vi "Autonomous Independent.vi"() -> ()   [LabVIEW 2016]
doc: "This VI is called when autonomous begins, and will automatically be terminated when autonomous ends. You can carry out timed or sensor driven robot movement independently without needing to return to the caller."
uses:
  <vilib>/Rock Robotics/WPI/Relay/WPI_RelayValue.ctl
  <vilib>/Rock Robotics/WPI/Utilities/WPI_GetSetVariantRefNum.vi
  <vilib>/Rock Robotics/Network Tables/NT Read String.vi
  <vilib>/Rock Robotics/Network Tables/NT Write Numeric Array.vi
  Robot Global Data.vi
  <vilib>/Rock Robotics/WPI/RobotDrive/WPI_RobotDriveArcadeDrive_Standard(NoSaturation).vi
  <vilib>/Rock Robotics/WPI/RobotDrive/WPI_RobotDriveArcadeDrive_RatioCurve.vi
panel:
  out "time up? 16":bool
  out "time up? 15":bool
  out "time up? 14":bool
  out "time up? 13":bool
  out "time up? 12":bool
  out "time up? 11":bool
  out "time up? 10":bool
  out "time up? 9":bool
  out "time up? 8":bool
  out "time up? 7":bool
  out "time up? 6":bool
  out "time up? 5":bool
  out "time up? 4":bool
  out "time up? 3":bool
  in  "Base 2":dbl=0.6
  in  "Tolerance 2":dbl=0.08
  in  "Ratio 2":dbl=0.25 format="%#_13g"
  out "time up? 2":bool
  out "time up?":bool
  in  "Ratio":dbl=0.25 format="%#_13g"
  in  "Tolerance":dbl=0.08
  in  "Base":dbl=0.6
  # "Be sure to right-click and choose Data Operations>>Make Current Value default if you want to save the array values with the VI"
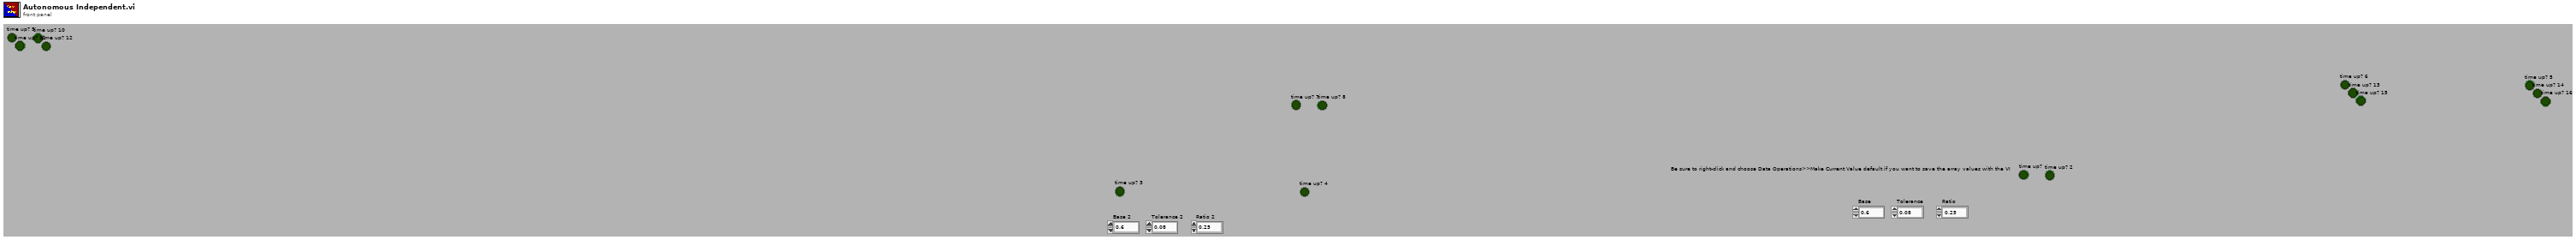
[diagram p1: front panel]
types:
  T1 = typedef "WPI_JoystickDevRef.ctl" = cluster{"Device":T2}
  T2 = typedef "WPI_JoystickDeviceEnum.ctl" = enum16{"USB 0", "USB 1", "USB 2", "USB 3", "USB 4", "USB 5"}
  T3 = typedef "WPI_RobotDriveDevRef.ctl" = cluster{"DevStatus":errorcluster, "Motors[]":T4[], "Square Inputs":bool, "Max Output":dbl}
  T4 = typedef "WPI_MotorControlDeviceRef.ctl" = cluster{"DeviceStatus":errorcluster, "Type":T5, "PWM":cluster{"PWM Channel":T6, "DeadBand":T7}, "CAN":cluster{"Device Number":u8, "SetOutput VI Ref":variant, "GetOutput VI Ref":variant, "Enable VI Ref":variant, "Disable VI Ref":variant, "Data":variant}, "Invert":bool}
  T5 = typedef "WPI_MotorControlType.ctl" = enum16{"PWM", "CAN"}
  T6 = typedef "FPGA_DIOPWMChannel.ctl" = enum8{"PWM 0", "PWM 1", "PWM 2", "PWM 3", "PWM 4", "PWM 5", "PWM 6", "PWM 7", "PWM 8", "PWM 9", "PWM MXP 0", "PWM MXP 1", "PWM MXP 2", "PWM MXP 3", "PWM MXP 4", "PWM MXP 5", "PWM MXP 6", "PWM MXP 7", "PWM MXP 8", "PWM MXP 9", "Invalid"}
  T7 = typedef "WPI_PWMDeadband.ctl" = cluster{"Name":string, "maxPositivePwm":i32, "minPositivePwm":i32, "centerPwm":i32, "maxNegativePwm":i32, "minNegativePwm":i32, "angularRange":u16}
  T8 = typedef "WPI_RelayDevRef.ctl" = cluster{"DevStatus":errorcluster, "Relay Channel":T9, "Relay Direction":T10}
  T9 = typedef "FPGA_DIORelayChannel.ctl" = enum8{"Relay 0", "Relay 1", "Relay 2", "Relay 3", "Invalid"}
  T10 = typedef "WPI_RelayDirection.ctl" = enum16{"Both directions", "Forward only", "Reverse only"}
  T11 = typedef "WPI_RelayValue.ctl" = enum16{"Off", "On", "Forward", "Reverse"}
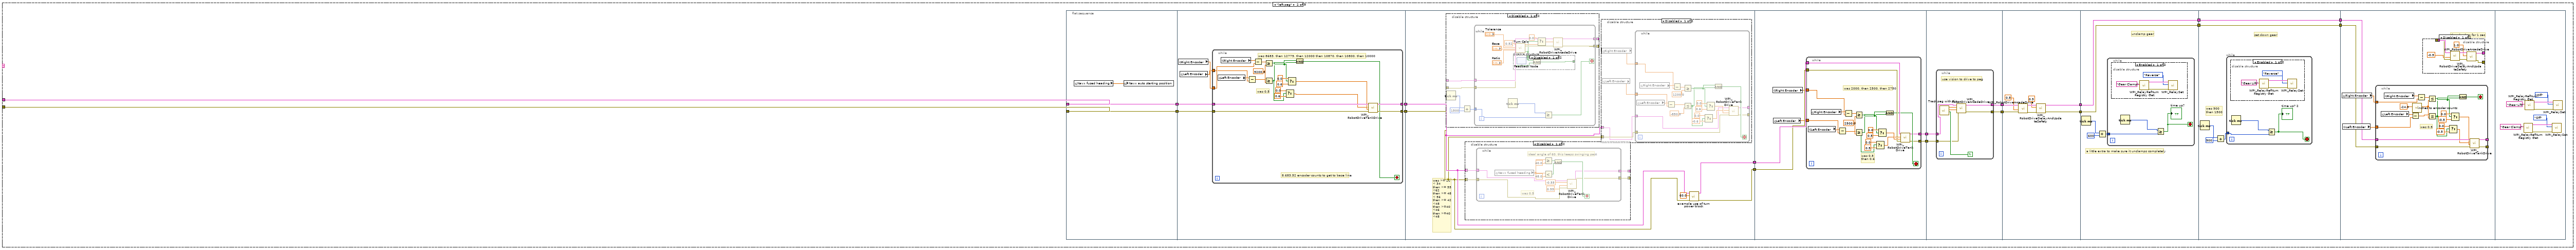
[diagram p3: hidden frame]
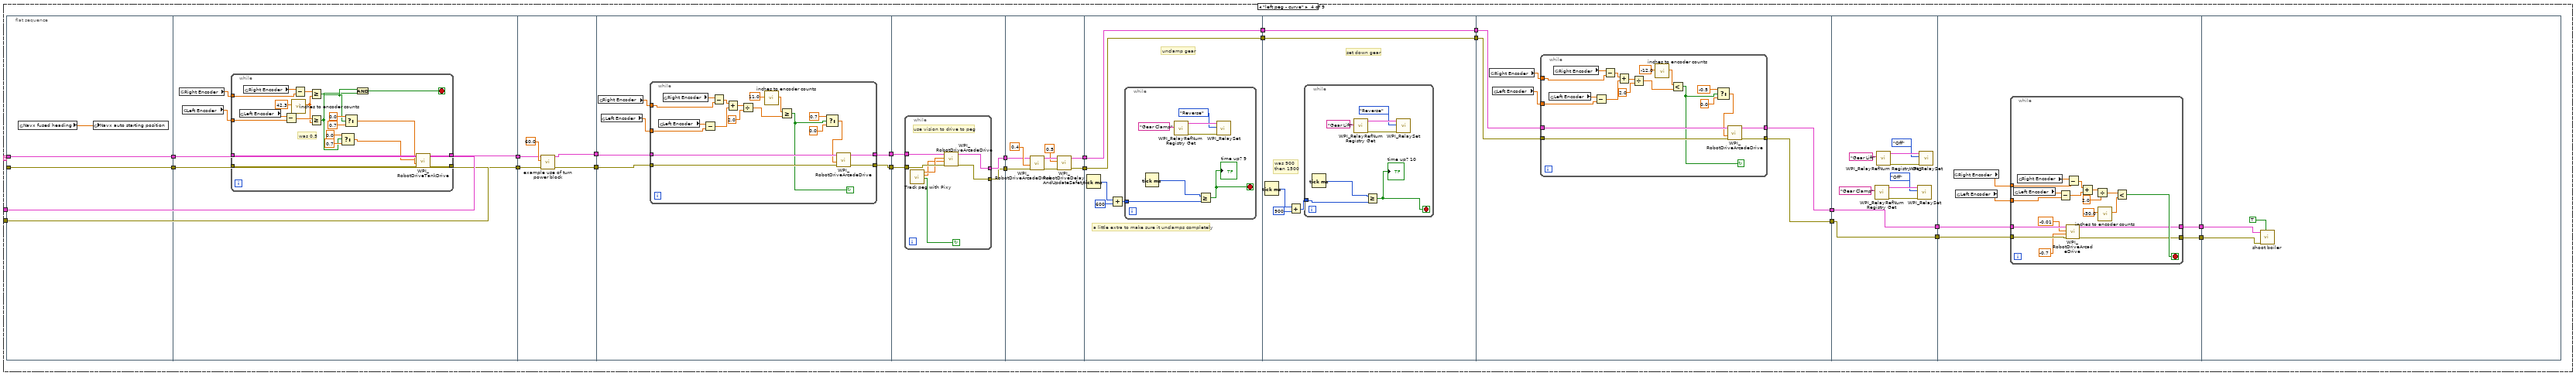
[diagram p14: hidden frame]
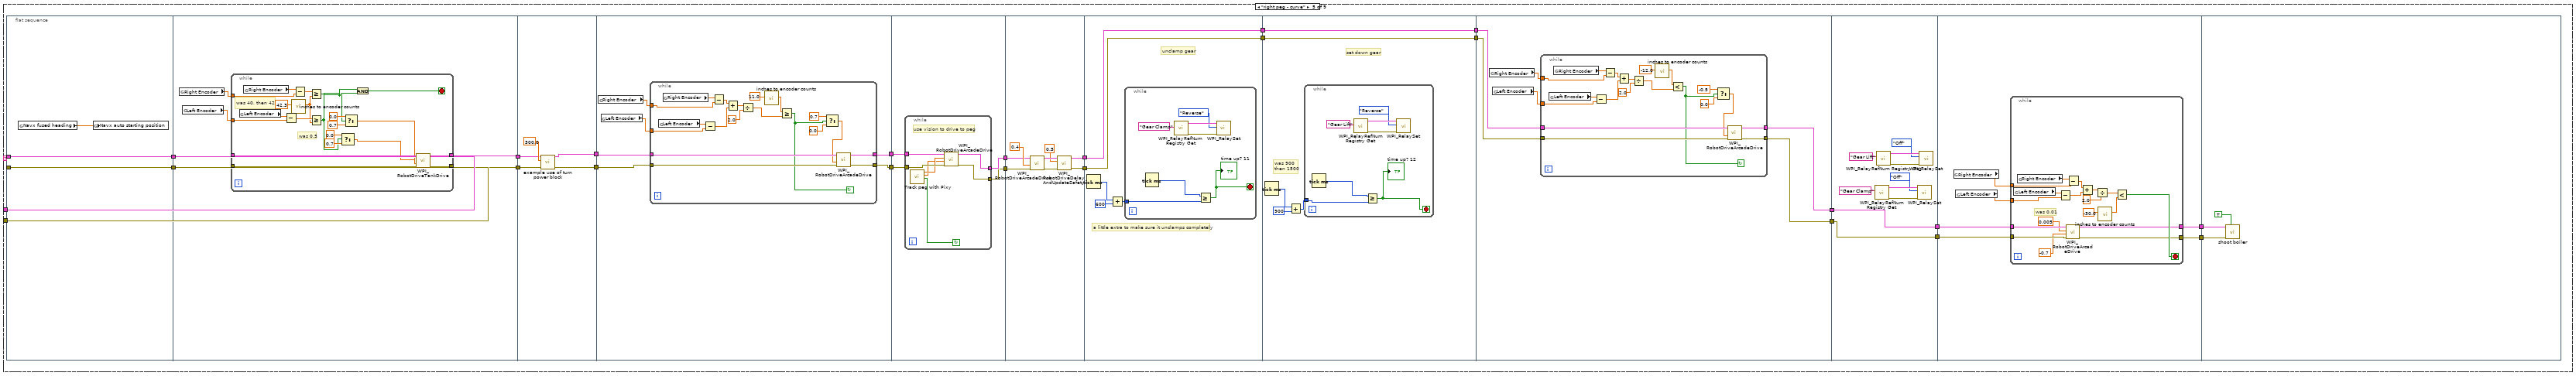
[diagram p15: hidden frame]
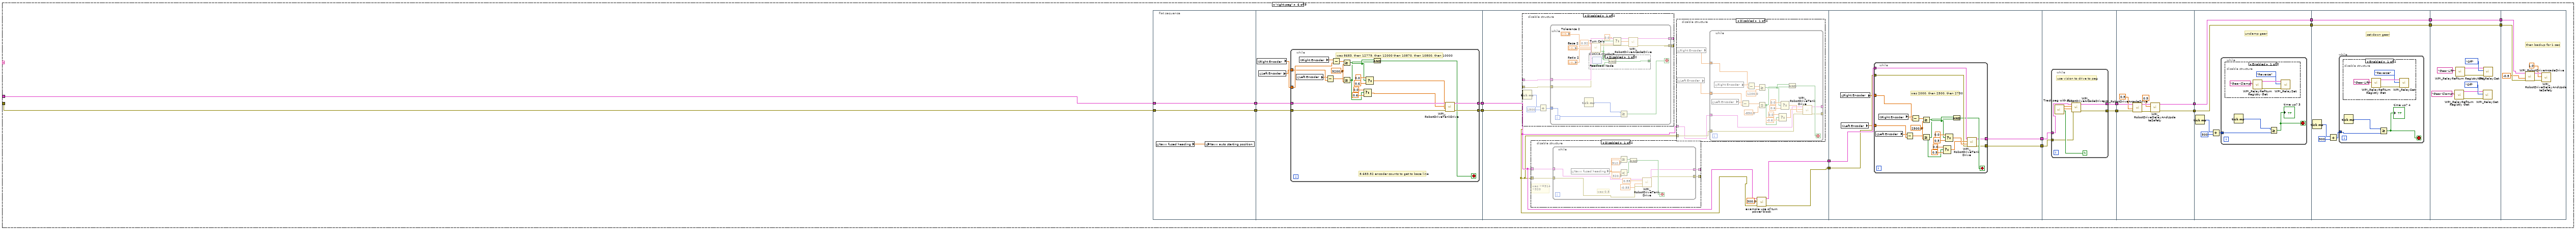
[diagram p16: hidden frame]
diagram:
  (unwired) "This function is run in parallel when the autonomous period begins. It will be terminated automatically when the period ends.\n\nNote that all Driver Station inputs are automatically latched and will not change once auto begins."
  # "This tells you the autonomous selected\nfrom the dashboard"
  # "Every 20ms, report that we are running autonomous\ncode. Loop will abort the same time as the VI."
  # "This gives you the joystick value\nthat is often the throttle"
  # "Use time and/or sensors to control how the robot drives."
  # "This tells you the driver position\nand alliance color"
  n1 = while {
    stop <- FALSE stop-if-true
    n2 = call <vilib>:"WPI_DriverStationReport Robot Code State.vi"("Autonomous"=TRUE) -> ()  [unwired: 10 in, 1 out]
    n3 = Wait (ms)(milliseconds to wait=u32 20) -> ()  [unwired: 1 out]
  }
  n4 = call <vilib>:"WPI_DriverStationGet Alliance Info.vi"() -> ()  [unwired: 12 out]
  n5 = call <vilib>:"WPI_JoystickRefNum Registry Get.vi"("refnum name"="Joystick 0") -> ("JoystickDevRef"=w15:T1)  [unwired: 1 in, 9 out]
  n6 = call <vilib>:"WPI_JoystickGetValues.vi"("JoystickDevRef"=w15) -> ("Axes"=w11:dbl[])  [unwired: 6 in, 4 out]
  n7 = call-poly <vilib>:"NT Read Value.vi"("Name"="Auto Selector") -> ("String"=w12:string)  [unwired: 9 in, 1 out]
  n8 = call-poly <vilib>:"NT Write Value.vi"("Numeric Array"=w11, "Name"="Joystick 0/Axes") -> ()  [unwired: 9 in, 1 out]
  n9 = Index Array(array=w11, index=2) -> ()  [unwired: 1 out]
  n10 = call <vilib>:"WPI_RobotDriveRefNum Registry Get.vi"("refnum name"="Drive") -> ("error out"=w7:errorcluster, "RobotDriveDevRef"=w8:T3)  [unwired: 9 in]
  n11 = call <vilib>:"WPI_RelayRefNum Registry Get.vi"("refnum name"="Ball Stirrer") -> ("error out"=w1:errorcluster, "RelayDevRef"=w2:T8)  [unwired: 9 in]
  n12 = call <vilib>:"WPI_MotorControlRefNum Registry Get.vi"("refnum name"="Shooter") -> ("error out"=w4:errorcluster, "MotorControlDevRef"=w5:T4)  [unwired: 9 in]
  n13 = case shown="\"center peg shoot - right\"" w12 {
    tunnel: w8 -> [_ w37 w257 w490 w679 w861 w1070 w1176 w1339]
    tunnel: w7 -> [_ w36 w256 w489 w678 w860 w1069 w1175 w1338]
    tunnel: w5 -> [_ _ _ _ _ _ _ _ _]
    tunnel: w4 -> [_ _ _ _ _ _ _ _ _]
    tunnel: w2 -> [_ _ _ _ _ _ _ _ _]
    tunnel: w1 -> [_ _ _ _ _ _ _ _ _]
    frame Default {
      # "You can put your main auto here, or you can right-click on the case and make any\nother frame be the default case."
      # "This is the frame that will execute if no selection is made, or if it is not recognized"
    }
    frame "left peg" {
      n14 = flat-sequence {
        tunnel: w36 -> [w39]
        tunnel: w37 -> [w40]
        tunnel: [w40] -> w21
        tunnel: [w39] -> w20
        tunnel: [w44] -> w27
        tunnel: [w43] -> w26
        tunnel: w21 -> [w46]
        tunnel: w20 -> [w45]
        tunnel: [w70] -> w25
        tunnel: w26 -> [w67]
        tunnel: w27 -> [w68]
        tunnel: [w69] -> w24
        tunnel: [w141] -> w35
        tunnel: [w140] -> w34
        tunnel: w25 -> [w143]
        tunnel: w24 -> [w142]
        tunnel: w35 -> [w167]
        tunnel: w34 -> [w166]
        tunnel: [w165] -> w31
        tunnel: [w164] -> w29
        tunnel: w31 -> [w182]
        tunnel: [w176] -> w30
        tunnel: w29 -> [w181]
        tunnel: [w175] -> w28
        tunnel: [w184] -> w33
        tunnel: w30 -> [w184]
        tunnel: [w183] -> w32
        tunnel: w28 -> [w183]
        tunnel: [w196] -> w23
        tunnel: w33 -> [w196]
        tunnel: [w195] -> w22
        tunnel: w32 -> [w195]
        tunnel: w22 -> [w207]
        tunnel: w23 -> [w208]
        frame #0 {
          n15 = global read "Robot Global Data.vi" "Navx fused heading"() -> (w38:dbl)
          n16 = global write "Robot Global Data.vi" "Navx auto starting position"(w38) -> ()
        }
        frame #1 {
          n17 = global read "Robot Global Data.vi" "Right Encoder"() -> (w42:dbl)
          n18 = global read "Robot Global Data.vi" "Left Encoder"() -> (w41:dbl)
          n19 = while {
            tunnel: w46 -> [w66]
            tunnel: w45 -> [w65]
            tunnel: [w57] -> w44
            tunnel: [w56] -> w43
            tunnel: w42 -> [w54]
            tunnel: w41 -> [w51]
            stop <- w49 stop-if-true
            w58 = 9200.0 ("y")
            # "was 0.5"
            # "was 8683, then 12779, then 12000 then 10870, then 10800, then 10000"
            # "8,683.52 encoder counts to get to base line"
            n20 = global read "Robot Global Data.vi" "Left Encoder"() -> (w52:dbl)
            n21 = global read "Robot Global Data.vi" "Right Encoder"() -> (w55:dbl)
            n22 = Subtract(x=w52, y=w51) -> (x-y=w50:dbl)
            n23 = Subtract(x=w55, y=w54) -> (x-y=w53:dbl)
            n24 = Greater Or Equal?(x=w53, y=w58) -> (x >= y?=w60:bool)
            n25 = Greater Or Equal?(x=w50, y=w58) -> (x >= y?=w59:bool)
            n26 = Select(t=0.0, s=w59, f=0.6) -> (s? t:f=w47:dbl)
            n27 = Select(t=0.0, s=w60, f=0.6) -> (s? t:f=w48:dbl)
            n28 = And(x=w60, y=w59) -> (x .and. y?=w49:bool)
            n29 = call <vilib>:"WPI_RobotDriveTankDrive.vi"("error in (no error)"=w65, "Right axis value"=w48, "Left axis value"=w47, "RobotDriveDevRef"=w66) -> ("error out"=w56:errorcluster, "RobotDriveDevRef"=w57:T3)  [unwired: 5 in, 1 out]
          }
        }
        frame #2 {
          # "was >= 28\n< 34\nthen >= 55\n<62\nthen >= 48\n< 56\nthen >= 42\n<48\nthen >=40\n<46\nthen >=40\n<48"
          n30 = disable-structure shown="Disabled" {
            disable-tunnel: _ -> [w119 _]
            disable-tunnel: _ -> [w118 _]
            disable-tunnel: [w117 _] -> _
            disable-tunnel: [w116 _] -> _
            frame Disabled {
              n31 = Tick Count (ms)() -> (millisecond timer value=w114:u32)
              n32 = Add(x=w114, y=u32 1500) -> (x+y=w113:u32)
              n33 = while {
                tunnel: w119 -> [w134]
                tunnel: w118 -> [w133]
                tunnel: [w124] -> w117
                tunnel: [w123] -> w116
                tunnel: w113 -> [w120]
                stop <- w121 stop-if-true
                n34 = Tick Count (ms)() -> (millisecond timer value=w122:u32)
                n35 = call "Turn Calc.vi"("Desired Angle (radians)"=0.52, "Tolerance"="Tolerance", "Base"="Base", "Ratio"="Ratio") -> ("Drive X Output"=w126:dbl, "In Range?"=w125:bool)  [unwired: 12 in, 2 out]
                n36 = disable-structure shown="Disabled" {
                  disable-tunnel: w125 -> [w136 _]
                  disable-tunnel: [w135 _] -> _
                  frame Disabled {
                    n37 = feedback #1() -> (w137:bool)  [unwired: 1 in]
                    n38 = feedback-in #1(w136) -> ()
                    n39 = And(x=w136, y=w137) -> (x .and. y?=w135:bool)
                  }
                  frame Enabled {
                  }
                }
                n40 = Select(t=0.0 ("f"), s=w125, f=w126) -> (s? t:f=w128:dbl)
                n41 = Greater Or Equal?(x=w122, y=w120) -> (x >= y?=w121:bool)
                n42 = call-poly <vilib>:"WPI_RobotDriveArcadeDrive.vi"("error in (no error)"=w133, "X axis value"=w128, "RobotDriveDevRef"=w134) -> ("error out"=w123:errorcluster, "RobotDriveDevRef"=w124:T3)  [unwired: 6 in, 1 out]
              }
            }
            frame Enabled {
            }
          }
          n43 = disable-structure shown="Disabled" {
            disable-tunnel: w67 -> [w75 _]
            disable-tunnel: w68 -> [w74 _]
            disable-tunnel: [w73 _] -> _
            disable-tunnel: [w72 _] -> _
            frame Disabled {
              n44 = while {
                tunnel: w74 -> [w76]
                tunnel: w75 -> [w80]
                tunnel: [w82] -> w73
                tunnel: [w81] -> w72
                stop <- w83 stop-if-true
                # "ideal angle of 60, this keeps swinging past"
                # "was 0.5"
                n45 = global read "Robot Global Data.vi" "Navx fused heading"() -> (w79:dbl)
                n46 = Greater Or Equal?(x=w79, y=40.0) -> (x >= y?=w85:bool)
                n47 = Less?(x=w79, y=48.0) -> (x < y?=w84:bool)
                n48 = And(x=w85, y=w84) -> (x .and. y?=w83:bool)
                n49 = call <vilib>:"WPI_RobotDriveTankDrive.vi"("error in (no error)"=w80, "Right axis value"=0.55, "Left axis value"=-0.55 ("x"), "RobotDriveDevRef"=w76) -> ("error out"=w81:errorcluster, "RobotDriveDevRef"=w82:T3)  [unwired: 5 in, 1 out]
              }
            }
            frame Enabled {
            }
          }
          n50 = disable-structure shown="Disabled" {
            disable-tunnel: w67 -> [w91 _]
            disable-tunnel: w68 -> [w90 _]
            frame Disabled {
              n51 = global read "Robot Global Data.vi" "Right Encoder"() -> (w88:dbl)
              n52 = global read "Robot Global Data.vi" "Left Encoder"() -> (w89:dbl)
              n53 = while {
                tunnel: w88 -> [w101]
                tunnel: w89 -> [w100]
                tunnel: [w96] -> _
                tunnel: [w95] -> _
                tunnel: w90 -> [w93]
                tunnel: w91 -> [w92]
                stop <- w97 stop-if-true
                n54 = global read "Robot Global Data.vi" "Left Encoder"() -> (w103:dbl)
                n55 = global read "Robot Global Data.vi" "Right Encoder"() -> (w105:dbl)
                n56 = Subtract(x=w103, y=w100) -> (x-y=w102:dbl)
                n57 = Subtract(x=w105, y=w101) -> (x-y=w104:dbl)
                n58 = Greater Or Equal?(x=w104, y=1200.0) -> (x >= y?=w108:bool)
                n59 = Less Or Equal?(x=w102, y=-850.0) -> (x <= y?=w107:bool)
                n60 = Select(t=0.0, s=w107, f=-0.6) -> (s? t:f=w98:dbl)
                n61 = Select(t=0.0, s=w108, f=0.6) -> (s? t:f=w99:dbl)
                n62 = And(x=w108, y=w107) -> (x .and. y?=w97:bool)
                n63 = call <vilib>:"WPI_RobotDriveTankDrive.vi"("error in (no error)"=w92, "Right axis value"=w99, "Left axis value"=w98, "RobotDriveDevRef"=w93) -> ("error out"=w95:errorcluster, "RobotDriveDevRef"=w96:T3)  [unwired: 5 in, 1 out]
              }
            }
            frame Enabled {
            }
          }
          n64 = call "example use of turn power block.vi"("error in (no error)"=w67, "desired angle"=60.0, "RobotDriveDevRef"=w68) -> ("error out"=w69:errorcluster, "RobotDriveDevRef 2"=w70:T3)  [unwired: 7 in]
        }
        frame #3 {
          n65 = global read "Robot Global Data.vi" "Right Encoder"() -> (w139:dbl)
          n66 = global read "Robot Global Data.vi" "Left Encoder"() -> (w138:dbl)
          n67 = while {
            tunnel: w139 -> [w152]
            tunnel: w138 -> [w151]
            tunnel: w143 -> [w148]
            tunnel: w142 -> [w147]
            tunnel: [w145] -> w141
            tunnel: [w144] -> w140
            stop <- w146 stop-if-true
            w157 = 2500.0 ("y")
            # "was 0.5\nthen 0.6"
            # "was 2000, then 2500, then 2750"
            n68 = global read "Robot Global Data.vi" "Left Encoder"() -> (w154:dbl)
            n69 = global read "Robot Global Data.vi" "Right Encoder"() -> (w156:dbl)
            n70 = Subtract(x=w154, y=w151) -> (x-y=w153:dbl)
            n71 = Subtract(x=w156, y=w152) -> (x-y=w155:dbl)
            n72 = Greater Or Equal?(x=w155, y=w157) -> (x >= y?=w159:bool)
            n73 = Greater Or Equal?(x=w153, y=w157) -> (x >= y?=w158:bool)
            n74 = Select(t=0.0, s=w158, f=0.5) -> (s? t:f=w149:dbl)
            n75 = Select(t=0.0, s=w159, f=0.5) -> (s? t:f=w150:dbl)
            n76 = And(x=w159, y=w158) -> (x .and. y?=w146:bool)
            n77 = call <vilib>:"WPI_RobotDriveTankDrive.vi"("error in (no error)"=w147, "Right axis value"=w150, "Left axis value"=w149, "RobotDriveDevRef"=w148) -> ("error out"=w144:errorcluster, "RobotDriveDevRef"=w145:T3)  [unwired: 5 in, 1 out]
          }
        }
        frame #4 {
          n78 = while {
            tunnel: w167 -> [w168]
            tunnel: w166 -> [w169]
            tunnel: [w171] -> w165
            tunnel: [w170] -> w164
            stop <- w172 continue-if-true
            # "use vision to drive to peg"
            n79 = call "Track peg with Pixy.vi"() -> ("sees peg"=w172:bool, "y output"=w173:dbl, "x output"=w174:dbl)  [unwired: 8 in]
            n80 = call-poly <vilib>:"WPI_RobotDriveArcadeDrive.vi"("error in (no error)"=w169, "Y axis value"=w173, "X axis value"=w174, "RobotDriveDevRef"=w168) -> ("error out"=w170:errorcluster, "RobotDriveDevRef"=w171:T3)  [unwired: 5 in, 1 out]
          }
        }
        frame #5 {
          n81 = call-poly <vilib>:"WPI_RobotDriveArcadeDrive.vi"("error in (no error)"=w181, "Y axis value"=0.5, "RobotDriveDevRef"=w182) -> ("error out"=w179:errorcluster, "RobotDriveDevRef"=w180:T3)  [unwired: 6 in, 1 out]
          n82 = call <vilib>:"WPI_RobotDriveDelayAndUpdateSafety.vi"("error in (no error)"=w179, "Delay (s)"=0.5, "RobotDriveDevRef"=w180) -> ("error out"=w175:errorcluster, "RobotDriveDevRef 2"=w176:T3)  [unwired: 7 in]
        }
        frame #6 {
          # "a little extra to make sure it unclamps completely"
          # "unclamp gear"
          n83 = Tick Count (ms)() -> (millisecond timer value=w186:u32)
          n84 = Add(x=w186, y=u32 600) -> (x+y=w185:u32)
          n85 = while {
            tunnel: w185 -> [w188]
            stop <- w189 stop-if-true
            n86 = disable-structure shown="Enabled" {
              frame Enabled {
                n87 = call <vilib>:"WPI_RelayRefNum Registry Get.vi"("refnum name"="Gear Clamp") -> ("error out"=w193:errorcluster, "RelayDevRef"=w194:T8)  [unwired: 9 in]
                n88 = call <vilib>:"WPI_RelaySet.vi"("error in (no error)"=w193, "RelayValue"=WPI_RelayValue."Reverse", "RelayDevRef"=w194) -> ()  [unwired: 7 in, 2 out]
              }
              frame Disabled {
              }
            }
            n89 = Tick Count (ms)() -> (millisecond timer value=w190:u32)
            n90 = Greater Or Equal?(x=w190, y=w188) -> (x >= y?=w189:bool)
            "time up?" <- w189
          }
        }
        frame #7 {
          # "was 900\nthen 1500"
          # "set down gear"
          n91 = Tick Count (ms)() -> (millisecond timer value=w199:u32)
          n92 = Add(x=w199, y=u32 900) -> (x+y=w197:u32)
          n93 = while {
            tunnel: w197 -> [w201]
            stop <- w200 stop-if-true
            n94 = disable-structure shown="Enabled" {
              frame Enabled {
                n95 = call <vilib>:"WPI_RelayRefNum Registry Get.vi"("refnum name"="Gear Lift") -> ("error out"=w205:errorcluster, "RelayDevRef"=w206:T8)  [unwired: 9 in]
                n96 = call <vilib>:"WPI_RelaySet.vi"("error in (no error)"=w205, "RelayValue"=WPI_RelayValue."Reverse", "RelayDevRef"=w206) -> ()  [unwired: 7 in, 2 out]
              }
              frame Disabled {
              }
            }
            n97 = Tick Count (ms)() -> (millisecond timer value=w202:u32)
            n98 = Greater Or Equal?(x=w202, y=w201) -> (x >= y?=w200:bool)
            "time up? 2" <- w200
          }
        }
        frame #8 {
          # "then backup for 1 sec"
          n99 = global read "Robot Global Data.vi" "Right Encoder"() -> (w210:dbl)
          n100 = global read "Robot Global Data.vi" "Left Encoder"() -> (w209:dbl)
          n101 = while {
            tunnel: w208 -> [w231]
            tunnel: w207 -> [w230]
            tunnel: [w223] -> _
            tunnel: [w222] -> _
            tunnel: w210 -> [w220]
            tunnel: w209 -> [w217]
            stop <- w216 stop-if-true
            # "was 0.5"
            n102 = global read "Robot Global Data.vi" "Left Encoder"() -> (w218:dbl)
            n103 = global read "Robot Global Data.vi" "Right Encoder"() -> (w221:dbl)
            n104 = Subtract(x=w218, y=w217) -> (x-y=w213:dbl)
            n105 = call "inches to encoder counts.vi"("x inches"=-24.0) -> ("encoder counts"=w212:dbl)  [unwired: 10 in]
            n106 = Subtract(x=w221, y=w220) -> (x-y=w219:dbl)
            n107 = Less Or Equal?(x=w219, y=w212) -> (x <= y?=w225:bool)
            n108 = Less Or Equal?(x=w213, y=w212) -> (x <= y?=w224:bool)
            n109 = Select(t=0.0, s=w224, f=-0.5) -> (s? t:f=w214:dbl)
            n110 = Select(t=0.0, s=w225, f=-0.5) -> (s? t:f=w215:dbl)
            n111 = And(x=w225, y=w224) -> (x .and. y?=w216:bool)
            n112 = call <vilib>:"WPI_RobotDriveTankDrive.vi"("error in (no error)"=w230, "Right axis value"=w215, "Left axis value"=w214, "RobotDriveDevRef"=w231) -> ("error out"=w222:errorcluster, "RobotDriveDevRef"=w223:T3)  [unwired: 5 in, 1 out]
          }
          n113 = disable-structure shown="Disabled" {
            disable-tunnel: _ -> [w239 _]
            disable-tunnel: _ -> [w238 _]
            disable-tunnel: [w233 _] -> _
            disable-tunnel: [w232 _] -> _
            frame Disabled {
              n114 = call-poly <vilib>:"WPI_RobotDriveArcadeDrive.vi"("error in (no error)"=w238, "Y axis value"=-0.5, "RobotDriveDevRef"=w239) -> ("error out"=w236:errorcluster, "RobotDriveDevRef"=w237:T3)  [unwired: 6 in, 1 out]
              n115 = call <vilib>:"WPI_RobotDriveDelayAndUpdateSafety.vi"("error in (no error)"=w236, "Delay (s)"=1.0, "RobotDriveDevRef"=w237) -> ("error out"=w232:errorcluster, "RobotDriveDevRef 2"=w233:T3)  [unwired: 7 in]
            }
            frame Enabled {
            }
          }
        }
        frame #9 {
          n116 = call <vilib>:"WPI_RelayRefNum Registry Get.vi"("refnum name"="Gear Clamp") -> ("error out"=w242:errorcluster, "RelayDevRef"=w243:T8)  [unwired: 9 in]
          n117 = call <vilib>:"WPI_RelayRefNum Registry Get.vi"("refnum name"="Gear Lift") -> ("error out"=w246:errorcluster, "RelayDevRef"=w247:T8)  [unwired: 9 in]
          n118 = call <vilib>:"WPI_RelaySet.vi"("error in (no error)"=w242, "RelayValue"=WPI_RelayValue."Off", "RelayDevRef"=w243) -> ()  [unwired: 7 in, 2 out]
          n119 = call <vilib>:"WPI_RelaySet.vi"("error in (no error)"=w246, "RelayValue"=WPI_RelayValue."Off", "RelayDevRef"=w247) -> ()  [unwired: 7 in, 2 out]
        }
      }
    }
    frame "left peg - shoot" {
      n120 = flat-sequence {
        tunnel: w256 -> [w275]
        tunnel: w257 -> [w276]
        tunnel: [w276] -> w273
        tunnel: [w275] -> w272
        tunnel: [w280] -> w270
        tunnel: [w279] -> w271
        tunnel: w273 -> [w282]
        tunnel: w272 -> [w281]
        tunnel: [w307] -> w269
        tunnel: w271 -> [w304]
        tunnel: w270 -> [w305]
        tunnel: [w306] -> w268
        tunnel: [w314] -> w267
        tunnel: [w313] -> w266
        tunnel: w269 -> [w310]
        tunnel: w268 -> [w309]
        tunnel: w267 -> [w338]
        tunnel: w266 -> [w337]
        tunnel: [w336] -> w265
        tunnel: [w335] -> w264
        tunnel: w265 -> [w353]
        tunnel: [w347] -> w263
        tunnel: w264 -> [w352]
        tunnel: [w346] -> w262
        tunnel: [w355] -> w261
        tunnel: w263 -> [w355]
        tunnel: [w354] -> w260
        tunnel: w262 -> [w354]
        tunnel: [w367] -> w258
        tunnel: w261 -> [w367]
        tunnel: [w366] -> w259
        tunnel: w260 -> [w366]
        tunnel: w259 -> [w380]
        tunnel: w258 -> [w381]
        tunnel: [w379] -> w254
        tunnel: [w378] -> w252
        tunnel: [w406] -> w255
        tunnel: w254 -> [w406]
        tunnel: [w405] -> w253
        tunnel: w252 -> [w405]
        tunnel: w255 -> [w418]
        tunnel: w253 -> [w417]
        tunnel: [w416] -> w251
        tunnel: [w415] -> w250
        tunnel: w251 -> [w423]
        tunnel: w250 -> [w422]
        tunnel: [w421] -> w249
        tunnel: [w420] -> w248
        tunnel: w249 -> [w448]
        tunnel: w248 -> [w447]
        frame #0 {
          n121 = global read "Robot Global Data.vi" "Navx fused heading"() -> (w274:dbl)
          n122 = global write "Robot Global Data.vi" "Navx auto starting position"(w274) -> ()
        }
        frame #1 {
          n123 = global read "Robot Global Data.vi" "Right Encoder"() -> (w278:dbl)
          n124 = global read "Robot Global Data.vi" "Left Encoder"() -> (w277:dbl)
          n125 = while {
            tunnel: w282 -> [w303]
            tunnel: w281 -> [w302]
            tunnel: [w295] -> w280
            tunnel: [w294] -> w279
            tunnel: w278 -> [w292]
            tunnel: w277 -> [w289]
            stop <- w287 stop-if-true
            # "was 0.5"
            # "was 8683, then 12779, then 12000 then 10870, then 10800, then 10000"
            n126 = global read "Robot Global Data.vi" "Left Encoder"() -> (w290:dbl)
            n127 = global read "Robot Global Data.vi" "Right Encoder"() -> (w293:dbl)
            n128 = Subtract(x=w290, y=w289) -> (x-y=w288:dbl)
            n129 = call "inches to encoder counts.vi"("x inches"=40.0) -> ("encoder counts"=w284:dbl)  [unwired: 10 in]
            n130 = Subtract(x=w293, y=w292) -> (x-y=w291:dbl)
            n131 = Greater Or Equal?(x=w291, y=w284) -> (x >= y?=w297:bool)
            n132 = Greater Or Equal?(x=w288, y=w284) -> (x >= y?=w296:bool)
            n133 = Select(t=0.0, s=w296, f=0.7) -> (s? t:f=w285:dbl)
            n134 = Select(t=0.0, s=w297, f=0.7) -> (s? t:f=w286:dbl)
            n135 = And(x=w297, y=w296) -> (x .and. y?=w287:bool)
            n136 = call <vilib>:"WPI_RobotDriveTankDrive.vi"("error in (no error)"=w302, "Right axis value"=w286, "Left axis value"=w285, "RobotDriveDevRef"=w303) -> ("error out"=w294:errorcluster, "RobotDriveDevRef"=w295:T3)  [unwired: 5 in, 1 out]
          }
        }
        frame #2 {
          # "was >= 28\n< 34\nthen >= 55\n<62\nthen >= 48\n< 56\nthen >= 42\n<48\nthen >=40\n<46\nthen >=40\n<48"
          n137 = call "example use of turn power block.vi"("error in (no error)"=w304, "desired angle"=60.0, "RobotDriveDevRef"=w305) -> ("error out"=w306:errorcluster, "RobotDriveDevRef 2"=w307:T3)  [unwired: 7 in]
        }
        frame #3 {
          n138 = global read "Robot Global Data.vi" "Right Encoder"() -> (w312:dbl)
          n139 = global read "Robot Global Data.vi" "Left Encoder"() -> (w311:dbl)
          n140 = while {
            tunnel: w312 -> [w323]
            tunnel: w311 -> [w322]
            tunnel: w310 -> [w319]
            tunnel: w309 -> [w318]
            tunnel: [w316] -> w314
            tunnel: [w315] -> w313
            stop <- w317 stop-if-true
            w328 = 2500.0 ("y")
            # "was 0.5\nthen 0.6"
            # "was 2000, then 2500, then 2750"
            n141 = global read "Robot Global Data.vi" "Left Encoder"() -> (w325:dbl)
            n142 = global read "Robot Global Data.vi" "Right Encoder"() -> (w327:dbl)
            n143 = Subtract(x=w325, y=w322) -> (x-y=w324:dbl)
            n144 = Subtract(x=w327, y=w323) -> (x-y=w326:dbl)
            n145 = Greater Or Equal?(x=w326, y=w328) -> (x >= y?=w330:bool)
            n146 = Greater Or Equal?(x=w324, y=w328) -> (x >= y?=w329:bool)
            n147 = Select(t=0.0, s=w329, f=0.7) -> (s? t:f=w320:dbl)
            n148 = Select(t=0.0, s=w330, f=0.7) -> (s? t:f=w321:dbl)
            n149 = And(x=w330, y=w329) -> (x .and. y?=w317:bool)
            n150 = call <vilib>:"WPI_RobotDriveTankDrive.vi"("error in (no error)"=w318, "Right axis value"=w321, "Left axis value"=w320, "RobotDriveDevRef"=w319) -> ("error out"=w315:errorcluster, "RobotDriveDevRef"=w316:T3)  [unwired: 5 in, 1 out]
          }
        }
        frame #4 {
          n151 = while {
            tunnel: w338 -> [w339]
            tunnel: w337 -> [w340]
            tunnel: [w342] -> w336
            tunnel: [w341] -> w335
            stop <- w343 continue-if-true
            # "use vision to drive to peg"
            n152 = call "Track peg with Pixy.vi"() -> ("sees peg"=w343:bool, "y output"=w344:dbl, "x output"=w345:dbl)  [unwired: 8 in]
            n153 = call-poly <vilib>:"WPI_RobotDriveArcadeDrive.vi"("error in (no error)"=w340, "Y axis value"=w344, "X axis value"=w345, "RobotDriveDevRef"=w339) -> ("error out"=w341:errorcluster, "RobotDriveDevRef"=w342:T3)  [unwired: 5 in, 1 out]
          }
        }
        frame #5 {
          n154 = call-poly <vilib>:"WPI_RobotDriveArcadeDrive.vi"("error in (no error)"=w352, "Y axis value"=0.5, "RobotDriveDevRef"=w353) -> ("error out"=w350:errorcluster, "RobotDriveDevRef"=w351:T3)  [unwired: 6 in, 1 out]
          n155 = call <vilib>:"WPI_RobotDriveDelayAndUpdateSafety.vi"("error in (no error)"=w350, "Delay (s)"=0.5, "RobotDriveDevRef"=w351) -> ("error out"=w346:errorcluster, "RobotDriveDevRef 2"=w347:T3)  [unwired: 7 in]
        }
        frame #6 {
          # "a little extra to make sure it unclamps completely"
          # "unclamp gear"
          n156 = Tick Count (ms)() -> (millisecond timer value=w357:u32)
          n157 = Add(x=w357, y=u32 600) -> (x+y=w356:u32)
          n158 = while {
            tunnel: w356 -> [w359]
            stop <- w360 stop-if-true
            n159 = disable-structure shown="Enabled" {
              frame Enabled {
                n160 = call <vilib>:"WPI_RelayRefNum Registry Get.vi"("refnum name"="Gear Clamp") -> ("error out"=w364:errorcluster, "RelayDevRef"=w365:T8)  [unwired: 9 in]
                n161 = call <vilib>:"WPI_RelaySet.vi"("error in (no error)"=w364, "RelayValue"=WPI_RelayValue."Reverse", "RelayDevRef"=w365) -> ()  [unwired: 7 in, 2 out]
              }
              frame Disabled {
              }
            }
            n162 = Tick Count (ms)() -> (millisecond timer value=w361:u32)
            n163 = Greater Or Equal?(x=w361, y=w359) -> (x >= y?=w360:bool)
            "time up? 7" <- w360
          }
        }
        frame #7 {
          # "was 900\nthen 1500"
          # "set down gear"
          n164 = Tick Count (ms)() -> (millisecond timer value=w370:u32)
          n165 = Add(x=w370, y=u32 900) -> (x+y=w368:u32)
          n166 = while {
            tunnel: w368 -> [w372]
            stop <- w371 stop-if-true
            n167 = disable-structure shown="Enabled" {
              frame Enabled {
                n168 = call <vilib>:"WPI_RelayRefNum Registry Get.vi"("refnum name"="Gear Lift") -> ("error out"=w376:errorcluster, "RelayDevRef"=w377:T8)  [unwired: 9 in]
                n169 = call <vilib>:"WPI_RelaySet.vi"("error in (no error)"=w376, "RelayValue"=WPI_RelayValue."Reverse", "RelayDevRef"=w377) -> ()  [unwired: 7 in, 2 out]
              }
              frame Disabled {
              }
            }
            n170 = Tick Count (ms)() -> (millisecond timer value=w373:u32)
            n171 = Greater Or Equal?(x=w373, y=w372) -> (x >= y?=w371:bool)
            "time up? 8" <- w371
          }
        }
        frame #8 {
          # "back away from peg"
          n172 = global read "Robot Global Data.vi" "Right Encoder"() -> (w383:dbl)
          n173 = global read "Robot Global Data.vi" "Left Encoder"() -> (w382:dbl)
          n174 = while {
            tunnel: w381 -> [w404]
            tunnel: w380 -> [w403]
            tunnel: [w396] -> w379
            tunnel: [w395] -> w378
            tunnel: w383 -> [w393]
            tunnel: w382 -> [w390]
            stop <- w389 stop-if-true
            # "was 0.5"
            n175 = global read "Robot Global Data.vi" "Left Encoder"() -> (w391:dbl)
            n176 = global read "Robot Global Data.vi" "Right Encoder"() -> (w394:dbl)
            n177 = Subtract(x=w391, y=w390) -> (x-y=w386:dbl)
            n178 = call "inches to encoder counts.vi"("x inches"=-24.0) -> ("encoder counts"=w385:dbl)  [unwired: 10 in]
            n179 = Subtract(x=w394, y=w393) -> (x-y=w392:dbl)
            n180 = Less Or Equal?(x=w392, y=w385) -> (x <= y?=w398:bool)
            n181 = Less Or Equal?(x=w386, y=w385) -> (x <= y?=w397:bool)
            n182 = Select(t=0.0, s=w397, f=-0.65) -> (s? t:f=w387:dbl)
            n183 = Select(t=0.0, s=w398, f=-0.65) -> (s? t:f=w388:dbl)
            n184 = And(x=w398, y=w397) -> (x .and. y?=w389:bool)
            n185 = call <vilib>:"WPI_RobotDriveTankDrive.vi"("error in (no error)"=w403, "Right axis value"=w388, "Left axis value"=w387, "RobotDriveDevRef"=w404) -> ("error out"=w395:errorcluster, "RobotDriveDevRef"=w396:T3)  [unwired: 5 in, 1 out]
          }
        }
        frame #9 {
          n186 = call <vilib>:"WPI_RelayRefNum Registry Get.vi"("refnum name"="Gear Clamp") -> ("error out"=w409:errorcluster, "RelayDevRef"=w410:T8)  [unwired: 9 in]
          n187 = call <vilib>:"WPI_RelayRefNum Registry Get.vi"("refnum name"="Gear Lift") -> ("error out"=w413:errorcluster, "RelayDevRef"=w414:T8)  [unwired: 9 in]
          n188 = call <vilib>:"WPI_RelaySet.vi"("error in (no error)"=w409, "RelayValue"=WPI_RelayValue."Off", "RelayDevRef"=w410) -> ()  [unwired: 7 in, 2 out]
          n189 = call <vilib>:"WPI_RelaySet.vi"("error in (no error)"=w413, "RelayValue"=WPI_RelayValue."Off", "RelayDevRef"=w414) -> ()  [unwired: 7 in, 2 out]
        }
        frame #10 {
          n190 = call "example use of turn power block.vi"("error in (no error)"=w417, "desired angle"=49.0, "RobotDriveDevRef"=w418) -> ("error out"=w415:errorcluster, "RobotDriveDevRef 2"=w416:T3)  [unwired: 7 in]
        }
        frame #11 {
          n191 = global read "Robot Global Data.vi" "Right Encoder"() -> (w425:dbl)
          n192 = global read "Robot Global Data.vi" "Left Encoder"() -> (w424:dbl)
          n193 = while {
            tunnel: w423 -> [w446]
            tunnel: w422 -> [w445]
            tunnel: [w439] -> w421
            tunnel: [w438] -> w420
            tunnel: w425 -> [w436]
            tunnel: w424 -> [w433]
            stop <- w432 stop-if-true
            # "was 0.5"
            n194 = global read "Robot Global Data.vi" "Left Encoder"() -> (w434:dbl)
            n195 = global read "Robot Global Data.vi" "Right Encoder"() -> (w437:dbl)
            n196 = Subtract(x=w434, y=w433) -> (x-y=w429:dbl)
            n197 = call "inches to encoder counts.vi"("x inches"=-35.0) -> ("encoder counts"=w428:dbl)  [unwired: 10 in]
            n198 = Subtract(x=w437, y=w436) -> (x-y=w435:dbl)
            n199 = Less Or Equal?(x=w435, y=w428) -> (x <= y?=w440:bool)
            n200 = Less Or Equal?(x=w429, y=w428) -> (x <= y?=w426:bool)
            n201 = Select(t=0.0, s=w426, f=-0.7) -> (s? t:f=w430:dbl)
            n202 = Select(t=0.0, s=w440, f=-0.7) -> (s? t:f=w431:dbl)
            n203 = And(x=w440, y=w426) -> (x .and. y?=w432:bool)
            n204 = call <vilib>:"WPI_RobotDriveTankDrive.vi"("error in (no error)"=w445, "Right axis value"=w431, "Left axis value"=w430, "RobotDriveDevRef"=w446) -> ("error out"=w438:errorcluster, "RobotDriveDevRef"=w439:T3)  [unwired: 5 in, 1 out]
          }
        }
        frame #12 {
          n205 = Tick Count (ms)() -> (millisecond timer value=w449:u32)
          n206 = while {
            tunnel: w449 -> [w457]
            tunnel: w448 -> [w451]
            tunnel: w447 -> [w450]
            stop <- w454 stop-if-true
            n207 = Tick Count (ms)() -> (millisecond timer value=w458:u32)
            n208 = Subtract(x=w458, y=w457) -> (x-y=w456:u32)
            n209 = Greater Or Equal?(x=w456, y=u32 800) -> (x >= y?=w454:bool)
            n210 = call "drive to boiler.vi"() -> ("y output"=w452:dbl, "x output"=w453:dbl)  [unwired: 10 in]
            n211 = call-poly <vilib>:"WPI_RobotDriveArcadeDrive.vi"("error in (no error)"=w450, "Y axis value"=w452, "X axis value"=w453, "RobotDriveDevRef"=w451) -> ()  [unwired: 5 in, 3 out]
          }
        }
        frame #13 {
          n212 = Tick Count (ms)() -> (millisecond timer value=w459:u32)
          n213 = while {
            tunnel: w459 -> [w464]
            stop <- FALSE stop-if-true
            # "was -0.8"
            n214 = Tick Count (ms)() -> (millisecond timer value=w466:u32)
            n215 = Subtract(x=w466, y=w464) -> (x-y=w463:u32)
            n216 = Greater Or Equal?(x=w463, y=u32 300) -> (x >= y?=w462:bool)
            n217 = call <vilib>:"WPI_RelayRefNum Registry Get.vi"("refnum name"="Ball Stirrer") -> ("error out"=w472:errorcluster, "RelayDevRef"=w471:T8)  [unwired: 9 in]
            n218 = Select(t=WPI_RelayValue."Reverse" ("RelayValue"), s=w462, f=WPI_RelayValue."Off" ("RelayValue")) -> (s? t:f=w470:T11)
            n219 = call <vilib>:"WPI_RelaySet.vi"("error in (no error)"=w472, "RelayValue"=w470, "RelayDevRef"=w471) -> ()  [unwired: 7 in, 2 out]
            n220 = call <vilib>:"WPI_MotorControlRefNum Registry Get.vi"("refnum name"="Shooter") -> ("error out"=w475:errorcluster, "MotorControlDevRef"=w474:T4)  [unwired: 9 in]
            n221 = call <vilib>:"WPI_MotorControlSetOutput.vi"("error in (no error)"=w475, "Output"=-0.75, "MotorControlDevRef"=w474) -> ()  [unwired: 6 in, 3 out]
          }
        }
        frame #14 {
        }
      }
    }
    frame "left peg - curve" {
      n222 = flat-sequence {
        tunnel: w489 -> [w501]
        tunnel: w490 -> [w502]
        tunnel: [w502] -> w499
        tunnel: [w501] -> w498
        tunnel: [w504] -> w497
        tunnel: w499 -> [w506]
        tunnel: w498 -> [w505]
        tunnel: [w503] -> w480
        tunnel: w497 -> [w533]
        tunnel: [w530] -> w479
        tunnel: [w531] -> w478
        tunnel: w480 -> [w532]
        tunnel: w479 -> [w538]
        tunnel: w478 -> [w537]
        tunnel: [w536] -> w477
        tunnel: [w535] -> w476
        tunnel: w477 -> [w562]
        tunnel: [w561] -> w488
        tunnel: [w560] -> w487
        tunnel: w476 -> [w563]
        tunnel: [w574] -> w496
        tunnel: [w573] -> w495
        tunnel: w488 -> [w572]
        tunnel: w487 -> [w571]
        tunnel: [w580] -> w494
        tunnel: w496 -> [w580]
        tunnel: [w579] -> w493
        tunnel: w495 -> [w579]
        tunnel: [w592] -> w491
        tunnel: w494 -> [w592]
        tunnel: [w591] -> w492
        tunnel: w493 -> [w591]
        tunnel: w492 -> [w605]
        tunnel: w491 -> [w606]
        tunnel: [w604] -> w485
        tunnel: [w603] -> w484
        tunnel: [w629] -> w486
        tunnel: w485 -> [w629]
        tunnel: w484 -> [w628]
        tunnel: [w628] -> w483
        tunnel: w486 -> [w641]
        tunnel: w483 -> [w640]
        tunnel: [w639] -> w482
        tunnel: [w638] -> w481
        tunnel: w482 -> [w663]
        tunnel: w481 -> [w662]
        frame #0 {
          n223 = global read "Robot Global Data.vi" "Navx fused heading"() -> (w500:dbl)
          n224 = global write "Robot Global Data.vi" "Navx auto starting position"(w500) -> ()
        }
        frame #1 {
          n225 = global read "Robot Global Data.vi" "Right Encoder"() -> (w508:dbl)
          n226 = global read "Robot Global Data.vi" "Left Encoder"() -> (w507:dbl)
          n227 = while {
            tunnel: w506 -> [w529]
            tunnel: w505 -> [w528]
            tunnel: [w521] -> w504
            tunnel: [w520] -> w503
            tunnel: w508 -> [w518]
            tunnel: w507 -> [w515]
            stop <- w513 stop-if-true
            # "was 0.5"
            n228 = global read "Robot Global Data.vi" "Left Encoder"() -> (w516:dbl)
            n229 = global read "Robot Global Data.vi" "Right Encoder"() -> (w519:dbl)
            n230 = Subtract(x=w516, y=w515) -> (x-y=w514:dbl)
            n231 = call "inches to encoder counts.vi"("x inches"=42.3) -> ("encoder counts"=w510:dbl)  [unwired: 10 in]
            n232 = Subtract(x=w519, y=w518) -> (x-y=w517:dbl)
            n233 = Greater Or Equal?(x=w517, y=w510) -> (x >= y?=w523:bool)
            n234 = Greater Or Equal?(x=w514, y=w510) -> (x >= y?=w522:bool)
            n235 = Select(t=0.0, s=w522, f=0.7) -> (s? t:f=w511:dbl)
            n236 = Select(t=0.0, s=w523, f=0.7) -> (s? t:f=w512:dbl)
            n237 = And(x=w523, y=w522) -> (x .and. y?=w513:bool)
            n238 = call <vilib>:"WPI_RobotDriveTankDrive.vi"("error in (no error)"=w528, "Right axis value"=w512, "Left axis value"=w511, "RobotDriveDevRef"=w529) -> ("error out"=w520:errorcluster, "RobotDriveDevRef"=w521:T3)  [unwired: 5 in, 1 out]
          }
        }
        frame #2 {
          n239 = call "example use of turn power block.vi"("error in (no error)"=w532, "desired angle"=60.0, "RobotDriveDevRef"=w533) -> ("error out"=w530:errorcluster, "RobotDriveDevRef 2"=w531:T3)  [unwired: 7 in]
        }
        frame #3 {
          n240 = global read "Robot Global Data.vi" "Right Encoder"() -> (w540:dbl)
          n241 = global read "Robot Global Data.vi" "Left Encoder"() -> (w539:dbl)
          n242 = while {
            tunnel: w537 -> [w559]
            tunnel: w538 -> [w558]
            tunnel: [w557] -> w536
            tunnel: [w556] -> w535
            tunnel: w540 -> [w554]
            tunnel: w539 -> [w552]
            stop <- w542 continue-if-true
            n243 = global read "Robot Global Data.vi" "Left Encoder"() -> (w553:dbl)
            n244 = global read "Robot Global Data.vi" "Right Encoder"() -> (w555:dbl)
            n245 = Subtract(x=w553, y=w552) -> (x-y=w549:dbl)
            n246 = Subtract(x=w555, y=w554) -> (x-y=w550:dbl)
            n247 = Add(x=w550, y=w549) -> (x+y=w548:dbl)
            n248 = Divide(x=w548, y=2.0) -> (x/y=w544:dbl)
            n249 = call "inches to encoder counts.vi"("x inches"=11.0) -> ("encoder counts"=w545:dbl)  [unwired: 10 in]
            n250 = Greater Or Equal?(x=w545, y=w544) -> (x >= y?=w542:bool)
            n251 = Select(t=0.7, s=w542, f=0.0) -> (s? t:f=w541:dbl)
            n252 = call-poly <vilib>:"WPI_RobotDriveArcadeDrive.vi"("error in (no error)"=w558, "Y axis value"=w541, "RobotDriveDevRef"=w559) -> ("error out"=w556:errorcluster, "RobotDriveDevRef"=w557:T3)  [unwired: 6 in, 1 out]
          }
        }
        frame #4 {
          n253 = while {
            tunnel: w563 -> [w568]
            tunnel: w562 -> [w569]
            tunnel: [w565] -> w561
            tunnel: [w564] -> w560
            stop <- w570 continue-if-true
            # "use vision to drive to peg"
            n254 = call "Track peg with Pixy.vi"() -> ("sees peg"=w570:bool, "y output"=w566:dbl, "x output"=w567:dbl)  [unwired: 8 in]
            n255 = call-poly <vilib>:"WPI_RobotDriveArcadeDrive.vi"("error in (no error)"=w568, "Y axis value"=w566, "X axis value"=w567, "RobotDriveDevRef"=w569) -> ("error out"=w564:errorcluster, "RobotDriveDevRef"=w565:T3)  [unwired: 5 in, 1 out]
          }
        }
        frame #5 {
          n256 = call-poly <vilib>:"WPI_RobotDriveArcadeDrive.vi"("error in (no error)"=w571, "Y axis value"=0.4, "RobotDriveDevRef"=w572) -> ("error out"=w577:errorcluster, "RobotDriveDevRef"=w578:T3)  [unwired: 6 in, 1 out]
          n257 = call <vilib>:"WPI_RobotDriveDelayAndUpdateSafety.vi"("error in (no error)"=w577, "Delay (s)"=0.5, "RobotDriveDevRef"=w578) -> ("error out"=w573:errorcluster, "RobotDriveDevRef 2"=w574:T3)  [unwired: 7 in]
        }
        frame #6 {
          # "a little extra to make sure it unclamps completely"
          # "unclamp gear"
          n258 = Tick Count (ms)() -> (millisecond timer value=w582:u32)
          n259 = Add(x=w582, y=u32 600) -> (x+y=w581:u32)
          n260 = while {
            tunnel: w581 -> [w588]
            stop <- w589 stop-if-true
            n261 = Tick Count (ms)() -> (millisecond timer value=w590:u32)
            n262 = call <vilib>:"WPI_RelayRefNum Registry Get.vi"("refnum name"="Gear Clamp") -> ("error out"=w586:errorcluster, "RelayDevRef"=w587:T8)  [unwired: 9 in]
            n263 = Greater Or Equal?(x=w590, y=w588) -> (x >= y?=w589:bool)
            "time up? 9" <- w589
            n264 = call <vilib>:"WPI_RelaySet.vi"("error in (no error)"=w586, "RelayValue"=WPI_RelayValue."Reverse", "RelayDevRef"=w587) -> ()  [unwired: 7 in, 2 out]
          }
        }
        frame #7 {
          # "was 900\nthen 1500"
          # "set down gear"
          n265 = Tick Count (ms)() -> (millisecond timer value=w595:u32)
          n266 = Add(x=w595, y=u32 900) -> (x+y=w593:u32)
          n267 = while {
            tunnel: w593 -> [w601]
            stop <- w600 stop-if-true
            n268 = Tick Count (ms)() -> (millisecond timer value=w602:u32)
            n269 = call <vilib>:"WPI_RelayRefNum Registry Get.vi"("refnum name"="Gear Lift") -> ("error out"=w598:errorcluster, "RelayDevRef"=w599:T8)  [unwired: 9 in]
            n270 = Greater Or Equal?(x=w602, y=w601) -> (x >= y?=w600:bool)
            "time up? 10" <- w600
            n271 = call <vilib>:"WPI_RelaySet.vi"("error in (no error)"=w598, "RelayValue"=WPI_RelayValue."Reverse", "RelayDevRef"=w599) -> ()  [unwired: 7 in, 2 out]
          }
        }
        frame #8 {
          n272 = global read "Robot Global Data.vi" "Right Encoder"() -> (w608:dbl)
          n273 = global read "Robot Global Data.vi" "Left Encoder"() -> (w607:dbl)
          n274 = while {
            tunnel: w606 -> [w627]
            tunnel: w605 -> [w626]
            tunnel: [w625] -> w604
            tunnel: [w624] -> w603
            tunnel: w608 -> [w622]
            tunnel: w607 -> [w620]
            stop <- w610 continue-if-true
            n275 = global read "Robot Global Data.vi" "Left Encoder"() -> (w621:dbl)
            n276 = global read "Robot Global Data.vi" "Right Encoder"() -> (w623:dbl)
            n277 = Subtract(x=w621, y=w620) -> (x-y=w617:dbl)
            n278 = Subtract(x=w623, y=w622) -> (x-y=w618:dbl)
            n279 = Add(x=w618, y=w617) -> (x+y=w616:dbl)
            n280 = Divide(x=w616, y=2.0) -> (x/y=w612:dbl)
            n281 = call "inches to encoder counts.vi"("x inches"=-12.0) -> ("encoder counts"=w613:dbl)  [unwired: 10 in]
            n282 = Less?(x=w613, y=w612) -> (x < y?=w610:bool)
            n283 = Select(t=-0.5, s=w610, f=0.0) -> (s? t:f=w609:dbl)
            n284 = call-poly <vilib>:"WPI_RobotDriveArcadeDrive.vi"("error in (no error)"=w626, "Y axis value"=w609, "RobotDriveDevRef"=w627) -> ("error out"=w624:errorcluster, "RobotDriveDevRef"=w625:T3)  [unwired: 6 in, 1 out]
          }
        }
        frame #9 {
          n285 = call <vilib>:"WPI_RelayRefNum Registry Get.vi"("refnum name"="Gear Clamp") -> ("error out"=w632:errorcluster, "RelayDevRef"=w633:T8)  [unwired: 9 in]
          n286 = call <vilib>:"WPI_RelayRefNum Registry Get.vi"("refnum name"="Gear Lift") -> ("error out"=w636:errorcluster, "RelayDevRef"=w637:T8)  [unwired: 9 in]
          n287 = call <vilib>:"WPI_RelaySet.vi"("error in (no error)"=w632, "RelayValue"=WPI_RelayValue."Off", "RelayDevRef"=w633) -> ()  [unwired: 7 in, 2 out]
          n288 = call <vilib>:"WPI_RelaySet.vi"("error in (no error)"=w636, "RelayValue"=WPI_RelayValue."Off", "RelayDevRef"=w637) -> ()  [unwired: 7 in, 2 out]
        }
        frame #10 {
          n289 = global read "Robot Global Data.vi" "Right Encoder"() -> (w643:dbl)
          n290 = global read "Robot Global Data.vi" "Left Encoder"() -> (w642:dbl)
          n291 = while {
            tunnel: w643 -> [w659]
            tunnel: w642 -> [w658]
            tunnel: w641 -> [w653]
            tunnel: w640 -> [w652]
            tunnel: [w645] -> w639
            tunnel: [w644] -> w638
            stop <- w649 stop-if-true
            n292 = global read "Robot Global Data.vi" "Left Encoder"() -> (w660:dbl)
            n293 = global read "Robot Global Data.vi" "Right Encoder"() -> (w661:dbl)
            n294 = Subtract(x=w660, y=w658) -> (x-y=w656:dbl)
            n295 = call-poly <vilib>:"WPI_RobotDriveArcadeDrive.vi"("error in (no error)"=w652, "Y axis value (Speed)"=-0.7, "X axis value (Curve)"=-0.01, "RobotDriveDevRef"=w653) -> ("error out"=w644:errorcluster, "RobotDriveDevRef"=w645:T3)  [unwired: 5 in, 1 out]
            n296 = Subtract(x=w661, y=w659) -> (x-y=w657:dbl)
            n297 = Add(x=w657, y=w656) -> (x+y=w655:dbl)
            n298 = Divide(x=w655, y=2.0) -> (x/y=w647:dbl)
            n299 = call "inches to encoder counts.vi"("x inches"=-30.0) -> ("encoder counts"=w646:dbl)  [unwired: 10 in]
            n300 = Less?(x=w647, y=w646) -> (x < y?=w649:bool)
          }
        }
        frame #11 {
          n301 = call "shoot boiler.vi"("go"=TRUE, "error out"=w662, "RobotDriveDevRef"=w663) -> ()  [unwired: 7 in, 2 out]
        }
      }
    }
    frame "right peg - curve" {
      n302 = flat-sequence {
        tunnel: w678 -> [w690]
        tunnel: w679 -> [w691]
        tunnel: [w691] -> w688
        tunnel: [w690] -> w687
        tunnel: [w693] -> w686
        tunnel: w688 -> [w695]
        tunnel: w687 -> [w694]
        tunnel: [w692] -> w669
        tunnel: w686 -> [w722]
        tunnel: [w719] -> w668
        tunnel: [w720] -> w667
        tunnel: w669 -> [w721]
        tunnel: w668 -> [w727]
        tunnel: w667 -> [w726]
        tunnel: [w725] -> w666
        tunnel: [w724] -> w665
        tunnel: w666 -> [w751]
        tunnel: [w750] -> w677
        tunnel: [w749] -> w676
        tunnel: w665 -> [w752]
        tunnel: [w763] -> w685
        tunnel: [w762] -> w684
        tunnel: w677 -> [w761]
        tunnel: w676 -> [w760]
        tunnel: [w769] -> w683
        tunnel: w685 -> [w769]
        tunnel: [w768] -> w682
        tunnel: w684 -> [w768]
        tunnel: [w781] -> w680
        tunnel: w683 -> [w781]
        tunnel: [w780] -> w681
        tunnel: w682 -> [w780]
        tunnel: w681 -> [w794]
        tunnel: w680 -> [w795]
        tunnel: [w793] -> w674
        tunnel: [w792] -> w673
        tunnel: [w818] -> w675
        tunnel: w674 -> [w818]
        tunnel: w673 -> [w817]
        tunnel: [w817] -> w672
        tunnel: w675 -> [w830]
        tunnel: w672 -> [w829]
        tunnel: [w828] -> w671
        tunnel: [w827] -> w670
        tunnel: w671 -> [w853]
        tunnel: w670 -> [w852]
        frame #0 {
          n303 = global read "Robot Global Data.vi" "Navx fused heading"() -> (w689:dbl)
          n304 = global write "Robot Global Data.vi" "Navx auto starting position"(w689) -> ()
        }
        frame #1 {
          n305 = global read "Robot Global Data.vi" "Right Encoder"() -> (w697:dbl)
          n306 = global read "Robot Global Data.vi" "Left Encoder"() -> (w696:dbl)
          n307 = while {
            tunnel: w695 -> [w718]
            tunnel: w694 -> [w717]
            tunnel: [w710] -> w693
            tunnel: [w709] -> w692
            tunnel: w697 -> [w707]
            tunnel: w696 -> [w704]
            stop <- w702 stop-if-true
            # "was 40, then 42"
            # "was 0.5"
            n308 = global read "Robot Global Data.vi" "Left Encoder"() -> (w705:dbl)
            n309 = global read "Robot Global Data.vi" "Right Encoder"() -> (w708:dbl)
            n310 = Subtract(x=w705, y=w704) -> (x-y=w703:dbl)
            n311 = call "inches to encoder counts.vi"("x inches"=42.3) -> ("encoder counts"=w699:dbl)  [unwired: 10 in]
            n312 = Subtract(x=w708, y=w707) -> (x-y=w706:dbl)
            n313 = Greater Or Equal?(x=w706, y=w699) -> (x >= y?=w712:bool)
            n314 = Greater Or Equal?(x=w703, y=w699) -> (x >= y?=w711:bool)
            n315 = Select(t=0.0, s=w711, f=0.7) -> (s? t:f=w700:dbl)
            n316 = Select(t=0.0, s=w712, f=0.7) -> (s? t:f=w701:dbl)
            n317 = And(x=w712, y=w711) -> (x .and. y?=w702:bool)
            n318 = call <vilib>:"WPI_RobotDriveTankDrive.vi"("error in (no error)"=w717, "Right axis value"=w701, "Left axis value"=w700, "RobotDriveDevRef"=w718) -> ("error out"=w709:errorcluster, "RobotDriveDevRef"=w710:T3)  [unwired: 5 in, 1 out]
          }
        }
        frame #2 {
          n319 = call "example use of turn power block.vi"("error in (no error)"=w721, "desired angle"=300.0, "RobotDriveDevRef"=w722) -> ("error out"=w719:errorcluster, "RobotDriveDevRef 2"=w720:T3)  [unwired: 7 in]
        }
        frame #3 {
          n320 = global read "Robot Global Data.vi" "Right Encoder"() -> (w729:dbl)
          n321 = global read "Robot Global Data.vi" "Left Encoder"() -> (w728:dbl)
          n322 = while {
            tunnel: w726 -> [w748]
            tunnel: w727 -> [w747]
            tunnel: [w746] -> w725
            tunnel: [w745] -> w724
            tunnel: w729 -> [w743]
            tunnel: w728 -> [w741]
            stop <- w731 continue-if-true
            n323 = global read "Robot Global Data.vi" "Left Encoder"() -> (w742:dbl)
            n324 = global read "Robot Global Data.vi" "Right Encoder"() -> (w744:dbl)
            n325 = Subtract(x=w742, y=w741) -> (x-y=w738:dbl)
            n326 = Subtract(x=w744, y=w743) -> (x-y=w739:dbl)
            n327 = Add(x=w739, y=w738) -> (x+y=w737:dbl)
            n328 = Divide(x=w737, y=2.0) -> (x/y=w733:dbl)
            n329 = call "inches to encoder counts.vi"("x inches"=11.0) -> ("encoder counts"=w734:dbl)  [unwired: 10 in]
            n330 = Greater Or Equal?(x=w734, y=w733) -> (x >= y?=w731:bool)
            n331 = Select(t=0.7, s=w731, f=0.0) -> (s? t:f=w730:dbl)
            n332 = call-poly <vilib>:"WPI_RobotDriveArcadeDrive.vi"("error in (no error)"=w747, "Y axis value"=w730, "RobotDriveDevRef"=w748) -> ("error out"=w745:errorcluster, "RobotDriveDevRef"=w746:T3)  [unwired: 6 in, 1 out]
          }
        }
        frame #4 {
          n333 = while {
            tunnel: w752 -> [w757]
            tunnel: w751 -> [w758]
            tunnel: [w754] -> w750
            tunnel: [w753] -> w749
            stop <- w759 continue-if-true
            # "use vision to drive to peg"
            n334 = call "Track peg with Pixy.vi"() -> ("sees peg"=w759:bool, "y output"=w755:dbl, "x output"=w756:dbl)  [unwired: 8 in]
            n335 = call-poly <vilib>:"WPI_RobotDriveArcadeDrive.vi"("error in (no error)"=w757, "Y axis value"=w755, "X axis value"=w756, "RobotDriveDevRef"=w758) -> ("error out"=w753:errorcluster, "RobotDriveDevRef"=w754:T3)  [unwired: 5 in, 1 out]
          }
        }
        frame #5 {
          n336 = call-poly <vilib>:"WPI_RobotDriveArcadeDrive.vi"("error in (no error)"=w760, "Y axis value"=0.4, "RobotDriveDevRef"=w761) -> ("error out"=w766:errorcluster, "RobotDriveDevRef"=w767:T3)  [unwired: 6 in, 1 out]
          n337 = call <vilib>:"WPI_RobotDriveDelayAndUpdateSafety.vi"("error in (no error)"=w766, "Delay (s)"=0.5, "RobotDriveDevRef"=w767) -> ("error out"=w762:errorcluster, "RobotDriveDevRef 2"=w763:T3)  [unwired: 7 in]
        }
        frame #6 {
          # "a little extra to make sure it unclamps completely"
          # "unclamp gear"
          n338 = Tick Count (ms)() -> (millisecond timer value=w771:u32)
          n339 = Add(x=w771, y=u32 600) -> (x+y=w770:u32)
          n340 = while {
            tunnel: w770 -> [w777]
            stop <- w778 stop-if-true
            n341 = Tick Count (ms)() -> (millisecond timer value=w779:u32)
            n342 = call <vilib>:"WPI_RelayRefNum Registry Get.vi"("refnum name"="Gear Clamp") -> ("error out"=w775:errorcluster, "RelayDevRef"=w776:T8)  [unwired: 9 in]
            n343 = Greater Or Equal?(x=w779, y=w777) -> (x >= y?=w778:bool)
            "time up? 11" <- w778
            n344 = call <vilib>:"WPI_RelaySet.vi"("error in (no error)"=w775, "RelayValue"=WPI_RelayValue."Reverse", "RelayDevRef"=w776) -> ()  [unwired: 7 in, 2 out]
          }
        }
        frame #7 {
          # "was 900\nthen 1500"
          # "set down gear"
          n345 = Tick Count (ms)() -> (millisecond timer value=w784:u32)
          n346 = Add(x=w784, y=u32 900) -> (x+y=w782:u32)
          n347 = while {
            tunnel: w782 -> [w790]
            stop <- w789 stop-if-true
            n348 = Tick Count (ms)() -> (millisecond timer value=w791:u32)
            n349 = call <vilib>:"WPI_RelayRefNum Registry Get.vi"("refnum name"="Gear Lift") -> ("error out"=w787:errorcluster, "RelayDevRef"=w788:T8)  [unwired: 9 in]
            n350 = Greater Or Equal?(x=w791, y=w790) -> (x >= y?=w789:bool)
            "time up? 12" <- w789
            n351 = call <vilib>:"WPI_RelaySet.vi"("error in (no error)"=w787, "RelayValue"=WPI_RelayValue."Reverse", "RelayDevRef"=w788) -> ()  [unwired: 7 in, 2 out]
          }
        }
        frame #8 {
          n352 = global read "Robot Global Data.vi" "Right Encoder"() -> (w797:dbl)
          n353 = global read "Robot Global Data.vi" "Left Encoder"() -> (w796:dbl)
          n354 = while {
            tunnel: w795 -> [w816]
            tunnel: w794 -> [w815]
            tunnel: [w814] -> w793
            tunnel: [w813] -> w792
            tunnel: w797 -> [w811]
            tunnel: w796 -> [w809]
            stop <- w799 continue-if-true
            n355 = global read "Robot Global Data.vi" "Left Encoder"() -> (w810:dbl)
            n356 = global read "Robot Global Data.vi" "Right Encoder"() -> (w812:dbl)
            n357 = Subtract(x=w810, y=w809) -> (x-y=w806:dbl)
            n358 = Subtract(x=w812, y=w811) -> (x-y=w807:dbl)
            n359 = Add(x=w807, y=w806) -> (x+y=w805:dbl)
            n360 = Divide(x=w805, y=2.0) -> (x/y=w801:dbl)
            n361 = call "inches to encoder counts.vi"("x inches"=-12.0) -> ("encoder counts"=w802:dbl)  [unwired: 10 in]
            n362 = Less?(x=w802, y=w801) -> (x < y?=w799:bool)
            n363 = Select(t=-0.5, s=w799, f=0.0) -> (s? t:f=w798:dbl)
            n364 = call-poly <vilib>:"WPI_RobotDriveArcadeDrive.vi"("error in (no error)"=w815, "Y axis value"=w798, "RobotDriveDevRef"=w816) -> ("error out"=w813:errorcluster, "RobotDriveDevRef"=w814:T3)  [unwired: 6 in, 1 out]
          }
        }
        frame #9 {
          n365 = call <vilib>:"WPI_RelayRefNum Registry Get.vi"("refnum name"="Gear Clamp") -> ("error out"=w821:errorcluster, "RelayDevRef"=w822:T8)  [unwired: 9 in]
          n366 = call <vilib>:"WPI_RelayRefNum Registry Get.vi"("refnum name"="Gear Lift") -> ("error out"=w825:errorcluster, "RelayDevRef"=w826:T8)  [unwired: 9 in]
          n367 = call <vilib>:"WPI_RelaySet.vi"("error in (no error)"=w821, "RelayValue"=WPI_RelayValue."Off", "RelayDevRef"=w822) -> ()  [unwired: 7 in, 2 out]
          n368 = call <vilib>:"WPI_RelaySet.vi"("error in (no error)"=w825, "RelayValue"=WPI_RelayValue."Off", "RelayDevRef"=w826) -> ()  [unwired: 7 in, 2 out]
        }
        frame #10 {
          n369 = global read "Robot Global Data.vi" "Right Encoder"() -> (w832:dbl)
          n370 = global read "Robot Global Data.vi" "Left Encoder"() -> (w831:dbl)
          n371 = while {
            tunnel: w832 -> [w848]
            tunnel: w831 -> [w847]
            tunnel: w830 -> [w842]
            tunnel: w829 -> [w841]
            tunnel: [w834] -> w828
            tunnel: [w833] -> w827
            stop <- w838 stop-if-true
            # "was 0.01"
            n372 = global read "Robot Global Data.vi" "Left Encoder"() -> (w849:dbl)
            n373 = global read "Robot Global Data.vi" "Right Encoder"() -> (w850:dbl)
            n374 = Subtract(x=w849, y=w847) -> (x-y=w845:dbl)
            n375 = call-poly <vilib>:"WPI_RobotDriveArcadeDrive.vi"("error in (no error)"=w841, "Y axis value (Speed)"=-0.7, "X axis value (Curve)"=0.005, "RobotDriveDevRef"=w842) -> ("error out"=w833:errorcluster, "RobotDriveDevRef"=w834:T3)  [unwired: 5 in, 1 out]
            n376 = Subtract(x=w850, y=w848) -> (x-y=w846:dbl)
            n377 = Add(x=w846, y=w845) -> (x+y=w844:dbl)
            n378 = Divide(x=w844, y=2.0) -> (x/y=w836:dbl)
            n379 = call "inches to encoder counts.vi"("x inches"=-30.0) -> ("encoder counts"=w835:dbl)  [unwired: 10 in]
            n380 = Less?(x=w836, y=w835) -> (x < y?=w838:bool)
          }
        }
        frame #11 {
          n381 = call "shoot boiler.vi"("go"=TRUE, "error out"=w852, "RobotDriveDevRef"=w853) -> ()  [unwired: 7 in, 2 out]
        }
      }
    }
    frame "right peg" {
      n382 = flat-sequence {
        tunnel: w860 -> [w875]
        tunnel: w861 -> [w876]
        tunnel: [w876] -> w855
        tunnel: [w875] -> w854
        tunnel: [w880] -> w873
        tunnel: [w879] -> w872
        tunnel: w855 -> [w882]
        tunnel: w854 -> [w881]
        tunnel: [w905] -> w871
        tunnel: [w906] -> w870
        tunnel: w872 -> [w903]
        tunnel: w873 -> [w904]
        tunnel: [w977] -> w869
        tunnel: [w976] -> w868
        tunnel: w870 -> [w979]
        tunnel: w871 -> [w978]
        tunnel: w869 -> [w1003]
        tunnel: w868 -> [w1002]
        tunnel: [w1001] -> w867
        tunnel: [w1000] -> w866
        tunnel: w867 -> [w1018]
        tunnel: [w1012] -> w865
        tunnel: w866 -> [w1017]
        tunnel: [w1011] -> w864
        tunnel: [w1020] -> w863
        tunnel: w865 -> [w1020]
        tunnel: [w1019] -> w862
        tunnel: w864 -> [w1019]
        tunnel: [w1032] -> w859
        tunnel: w863 -> [w1032]
        tunnel: [w1031] -> w857
        tunnel: w862 -> [w1031]
        tunnel: w859 -> [w1052]
        tunnel: [w1052] -> w858
        tunnel: w857 -> [w1051]
        tunnel: [w1051] -> w856
        tunnel: w858 -> [w1058]
        tunnel: w856 -> [w1057]
        frame #0 {
          n383 = global read "Robot Global Data.vi" "Navx fused heading"() -> (w874:dbl)
          n384 = global write "Robot Global Data.vi" "Navx auto starting position"(w874) -> ()
        }
        frame #1 {
          n385 = global read "Robot Global Data.vi" "Right Encoder"() -> (w878:dbl)
          n386 = global read "Robot Global Data.vi" "Left Encoder"() -> (w877:dbl)
          n387 = while {
            tunnel: w882 -> [w902]
            tunnel: w881 -> [w901]
            tunnel: [w893] -> w880
            tunnel: [w892] -> w879
            tunnel: w878 -> [w890]
            tunnel: w877 -> [w887]
            stop <- w885 stop-if-true
            w894 = 9200.0 ("y")
            # "was 8683, then 12779, then 12000 then 10870, then 10800, then 10000"
            # "8,683.52 encoder counts to get to base line"
            n388 = global read "Robot Global Data.vi" "Left Encoder"() -> (w888:dbl)
            n389 = global read "Robot Global Data.vi" "Right Encoder"() -> (w891:dbl)
            n390 = Subtract(x=w888, y=w887) -> (x-y=w886:dbl)
            n391 = Subtract(x=w891, y=w890) -> (x-y=w889:dbl)
            n392 = Greater Or Equal?(x=w889, y=w894) -> (x >= y?=w896:bool)
            n393 = Greater Or Equal?(x=w886, y=w894) -> (x >= y?=w895:bool)
            n394 = Select(t=0.0, s=w895, f=0.6) -> (s? t:f=w883:dbl)
            n395 = Select(t=0.0, s=w896, f=0.6) -> (s? t:f=w884:dbl)
            n396 = And(x=w896, y=w895) -> (x .and. y?=w885:bool)
            n397 = call <vilib>:"WPI_RobotDriveTankDrive.vi"("error in (no error)"=w901, "Right axis value"=w884, "Left axis value"=w883, "RobotDriveDevRef"=w902) -> ("error out"=w892:errorcluster, "RobotDriveDevRef"=w893:T3)  [unwired: 5 in, 1 out]
          }
        }
        frame #2 {
          n398 = disable-structure shown="Disabled" {
            disable-tunnel: _ -> [w955 _]
            disable-tunnel: _ -> [w954 _]
            disable-tunnel: [w953 _] -> _
            disable-tunnel: [w952 _] -> _
            frame Disabled {
              n399 = Tick Count (ms)() -> (millisecond timer value=w950:u32)
              n400 = Add(x=w950, y=u32 1500) -> (x+y=w949:u32)
              n401 = while {
                tunnel: w955 -> [w970]
                tunnel: w954 -> [w969]
                tunnel: [w960] -> w953
                tunnel: [w959] -> w952
                tunnel: w949 -> [w956]
                stop <- w957 stop-if-true
                n402 = Tick Count (ms)() -> (millisecond timer value=w958:u32)
                n403 = call "Turn Calc.vi"("Desired Angle (radians)"=0.52, "Tolerance"="Tolerance 2", "Base"="Base 2", "Ratio"="Ratio 2") -> ("Drive X Output"=w962:dbl, "In Range?"=w961:bool)  [unwired: 12 in, 2 out]
                n404 = disable-structure shown="Disabled" {
                  disable-tunnel: w961 -> [w972 _]
                  disable-tunnel: [w971 _] -> _
                  frame Disabled {
                    n405 = feedback #2() -> (w973:bool)  [unwired: 1 in]
                    n406 = feedback-in #2(w972) -> ()
                    n407 = And(x=w972, y=w973) -> (x .and. y?=w971:bool)
                  }
                  frame Enabled {
                  }
                }
                n408 = Select(t=0.0 ("f"), s=w961, f=w962) -> (s? t:f=w964:dbl)
                n409 = Greater Or Equal?(x=w958, y=w956) -> (x >= y?=w957:bool)
                n410 = call-poly <vilib>:"WPI_RobotDriveArcadeDrive.vi"("error in (no error)"=w969, "X axis value"=w964, "RobotDriveDevRef"=w970) -> ("error out"=w959:errorcluster, "RobotDriveDevRef"=w960:T3)  [unwired: 6 in, 1 out]
              }
            }
            frame Enabled {
            }
          }
          n411 = disable-structure shown="Disabled" {
            disable-tunnel: w903 -> [w911 _]
            disable-tunnel: w904 -> [w910 _]
            disable-tunnel: [w909 _] -> _
            disable-tunnel: [w908 _] -> _
            frame Disabled {
              # "was >=314\n<320"
              n412 = while {
                tunnel: w910 -> [w912]
                tunnel: w911 -> [w916]
                tunnel: [w918] -> w909
                tunnel: [w917] -> w908
                stop <- w919 stop-if-true
                # "was 0.5"
                n413 = global read "Robot Global Data.vi" "Navx fused heading"() -> (w915:dbl)
                n414 = Greater Or Equal?(x=w915, y=312.0) -> (x >= y?=w921:bool)
                n415 = Less?(x=w915, y=320.0) -> (x < y?=w920:bool)
                n416 = And(x=w921, y=w920) -> (x .and. y?=w919:bool)
                n417 = call <vilib>:"WPI_RobotDriveTankDrive.vi"("error in (no error)"=w916, "Right axis value"=-0.55, "Left axis value"=0.55 ("x"), "RobotDriveDevRef"=w912) -> ("error out"=w917:errorcluster, "RobotDriveDevRef"=w918:T3)  [unwired: 5 in, 1 out]
              }
            }
            frame Enabled {
            }
          }
          n418 = disable-structure shown="Disabled" {
            disable-tunnel: w903 -> [w927 _]
            disable-tunnel: w904 -> [w926 _]
            frame Disabled {
              n419 = global read "Robot Global Data.vi" "Right Encoder"() -> (w924:dbl)
              n420 = global read "Robot Global Data.vi" "Left Encoder"() -> (w925:dbl)
              n421 = while {
                tunnel: w924 -> [w937]
                tunnel: w925 -> [w936]
                tunnel: [w932] -> _
                tunnel: [w931] -> _
                tunnel: w926 -> [w929]
                tunnel: w927 -> [w928]
                stop <- w933 stop-if-true
                n422 = global read "Robot Global Data.vi" "Left Encoder"() -> (w939:dbl)
                n423 = global read "Robot Global Data.vi" "Right Encoder"() -> (w941:dbl)
                n424 = Subtract(x=w939, y=w936) -> (x-y=w938:dbl)
                n425 = Subtract(x=w941, y=w937) -> (x-y=w940:dbl)
                n426 = Greater Or Equal?(x=w940, y=1200.0) -> (x >= y?=w944:bool)
                n427 = Less Or Equal?(x=w938, y=-850.0) -> (x <= y?=w943:bool)
                n428 = Select(t=0.0, s=w943, f=-0.6) -> (s? t:f=w934:dbl)
                n429 = Select(t=0.0, s=w944, f=0.6) -> (s? t:f=w935:dbl)
                n430 = And(x=w944, y=w943) -> (x .and. y?=w933:bool)
                n431 = call <vilib>:"WPI_RobotDriveTankDrive.vi"("error in (no error)"=w928, "Right axis value"=w935, "Left axis value"=w934, "RobotDriveDevRef"=w929) -> ("error out"=w931:errorcluster, "RobotDriveDevRef"=w932:T3)  [unwired: 5 in, 1 out]
              }
            }
            frame Enabled {
            }
          }
          n432 = call "example use of turn power block.vi"("error in (no error)"=w903, "desired angle"=300.0, "RobotDriveDevRef"=w904) -> ("error out"=w905:errorcluster, "RobotDriveDevRef 2"=w906:T3)  [unwired: 7 in]
        }
        frame #3 {
          n433 = global read "Robot Global Data.vi" "Right Encoder"() -> (w975:dbl)
          n434 = global read "Robot Global Data.vi" "Left Encoder"() -> (w974:dbl)
          n435 = while {
            tunnel: w975 -> [w988]
            tunnel: w974 -> [w987]
            tunnel: w979 -> [w984]
            tunnel: w978 -> [w983]
            tunnel: [w981] -> w977
            tunnel: [w980] -> w976
            stop <- w982 stop-if-true
            w993 = 2500.0 ("y")
            # "was 2000, then 2500, then 2750"
            n436 = global read "Robot Global Data.vi" "Left Encoder"() -> (w990:dbl)
            n437 = global read "Robot Global Data.vi" "Right Encoder"() -> (w992:dbl)
            n438 = Subtract(x=w990, y=w987) -> (x-y=w989:dbl)
            n439 = Subtract(x=w992, y=w988) -> (x-y=w991:dbl)
            n440 = Greater Or Equal?(x=w991, y=w993) -> (x >= y?=w995:bool)
            n441 = Greater Or Equal?(x=w989, y=w993) -> (x >= y?=w994:bool)
            n442 = Select(t=0.0, s=w994, f=0.5) -> (s? t:f=w985:dbl)
            n443 = Select(t=0.0, s=w995, f=0.5) -> (s? t:f=w986:dbl)
            n444 = And(x=w995, y=w994) -> (x .and. y?=w982:bool)
            n445 = call <vilib>:"WPI_RobotDriveTankDrive.vi"("error in (no error)"=w983, "Right axis value"=w986, "Left axis value"=w985, "RobotDriveDevRef"=w984) -> ("error out"=w980:errorcluster, "RobotDriveDevRef"=w981:T3)  [unwired: 5 in, 1 out]
          }
        }
        frame #4 {
          n446 = while {
            tunnel: w1003 -> [w1004]
            tunnel: w1002 -> [w1005]
            tunnel: [w1007] -> w1001
            tunnel: [w1006] -> w1000
            stop <- w1008 continue-if-true
            # "use vision to drive to peg"
            n447 = call "Track peg with Pixy.vi"() -> ("sees peg"=w1008:bool, "y output"=w1009:dbl, "x output"=w1010:dbl)  [unwired: 8 in]
            n448 = call-poly <vilib>:"WPI_RobotDriveArcadeDrive.vi"("error in (no error)"=w1005, "Y axis value"=w1009, "X axis value"=w1010, "RobotDriveDevRef"=w1004) -> ("error out"=w1006:errorcluster, "RobotDriveDevRef"=w1007:T3)  [unwired: 5 in, 1 out]
          }
        }
        frame #5 {
          n449 = call-poly <vilib>:"WPI_RobotDriveArcadeDrive.vi"("error in (no error)"=w1017, "Y axis value"=0.5, "RobotDriveDevRef"=w1018) -> ("error out"=w1015:errorcluster, "RobotDriveDevRef"=w1016:T3)  [unwired: 6 in, 1 out]
          n450 = call <vilib>:"WPI_RobotDriveDelayAndUpdateSafety.vi"("error in (no error)"=w1015, "Delay (s)"=0.5, "RobotDriveDevRef"=w1016) -> ("error out"=w1011:errorcluster, "RobotDriveDevRef 2"=w1012:T3)  [unwired: 7 in]
        }
        frame #6 {
          # "unclamp gear"
          n451 = Tick Count (ms)() -> (millisecond timer value=w1022:u32)
          n452 = Add(x=w1022, y=u32 500) -> (x+y=w1021:u32)
          n453 = while {
            tunnel: w1021 -> [w1024]
            stop <- w1025 stop-if-true
            n454 = disable-structure shown="Enabled" {
              frame Enabled {
                n455 = call <vilib>:"WPI_RelayRefNum Registry Get.vi"("refnum name"="Gear Clamp") -> ("error out"=w1029:errorcluster, "RelayDevRef"=w1030:T8)  [unwired: 9 in]
                n456 = call <vilib>:"WPI_RelaySet.vi"("error in (no error)"=w1029, "RelayValue"=WPI_RelayValue."Reverse", "RelayDevRef"=w1030) -> ()  [unwired: 7 in, 2 out]
              }
              frame Disabled {
              }
            }
            n457 = Tick Count (ms)() -> (millisecond timer value=w1026:u32)
            n458 = Greater Or Equal?(x=w1026, y=w1024) -> (x >= y?=w1025:bool)
            "time up? 3" <- w1025
          }
        }
        frame #7 {
          # "set down gear"
          n459 = Tick Count (ms)() -> (millisecond timer value=w1035:u32)
          n460 = Add(x=w1035, y=u32 900) -> (x+y=w1033:u32)
          n461 = while {
            tunnel: w1033 -> [w1037]
            stop <- w1036 stop-if-true
            n462 = disable-structure shown="Enabled" {
              frame Enabled {
                n463 = call <vilib>:"WPI_RelayRefNum Registry Get.vi"("refnum name"="Gear Lift") -> ("error out"=w1041:errorcluster, "RelayDevRef"=w1042:T8)  [unwired: 9 in]
                n464 = call <vilib>:"WPI_RelaySet.vi"("error in (no error)"=w1041, "RelayValue"=WPI_RelayValue."Reverse", "RelayDevRef"=w1042) -> ()  [unwired: 7 in, 2 out]
              }
              frame Disabled {
              }
            }
            n465 = Tick Count (ms)() -> (millisecond timer value=w1038:u32)
            n466 = Greater Or Equal?(x=w1038, y=w1037) -> (x >= y?=w1036:bool)
            "time up? 4" <- w1036
          }
        }
        frame #8 {
          n467 = call <vilib>:"WPI_RelayRefNum Registry Get.vi"("refnum name"="Gear Clamp") -> ("error out"=w1044:errorcluster, "RelayDevRef"=w1043:T8)  [unwired: 9 in]
          n468 = call <vilib>:"WPI_RelayRefNum Registry Get.vi"("refnum name"="Gear Lift") -> ("error out"=w1048:errorcluster, "RelayDevRef"=w1047:T8)  [unwired: 9 in]
          n469 = call <vilib>:"WPI_RelaySet.vi"("error in (no error)"=w1044, "RelayValue"=WPI_RelayValue."Off", "RelayDevRef"=w1043) -> ()  [unwired: 7 in, 2 out]
          n470 = call <vilib>:"WPI_RelaySet.vi"("error in (no error)"=w1048, "RelayValue"=WPI_RelayValue."Off", "RelayDevRef"=w1047) -> ()  [unwired: 7 in, 2 out]
        }
        frame #9 {
          # "then backup for 1 sec"
          n471 = call-poly <vilib>:"WPI_RobotDriveArcadeDrive.vi"("error in (no error)"=w1057, "Y axis value"=-0.5, "RobotDriveDevRef"=w1058) -> ("error out"=w1055:errorcluster, "RobotDriveDevRef"=w1056:T3)  [unwired: 6 in, 1 out]
          n472 = call <vilib>:"WPI_RobotDriveDelayAndUpdateSafety.vi"("error in (no error)"=w1055, "Delay (s)"=1.0, "RobotDriveDevRef"=w1056) -> ()  [unwired: 7 in, 2 out]
        }
      }
    }
    frame "center peg" {
      n473 = flat-sequence {
        tunnel: w1069 -> [w1073]
        tunnel: w1070 -> [w1074]
        tunnel: [w1072] -> w1060
        tunnel: [w1071] -> w1059
        tunnel: [w1099] -> w1062
        tunnel: [w1098] -> w1061
        tunnel: w1060 -> [w1101]
        tunnel: w1059 -> [w1100]
        tunnel: [w1111] -> w1068
        tunnel: [w1110] -> w1067
        tunnel: w1061 -> [w1112]
        tunnel: w1062 -> [w1113]
        tunnel: w1068 -> [w1117]
        tunnel: w1067 -> [w1121]
        tunnel: [w1117] -> w1066
        tunnel: [w1121] -> w1065
        tunnel: w1066 -> [w1133]
        tunnel: w1065 -> [w1132]
        tunnel: [w1133] -> w1064
        tunnel: [w1132] -> w1063
        tunnel: w1064 -> [w1142]
        tunnel: w1063 -> [w1141]
        frame #0 {
          n474 = global read "Robot Global Data.vi" "Right Encoder"() -> (w1076:dbl)
          n475 = global read "Robot Global Data.vi" "Left Encoder"() -> (w1075:dbl)
          n476 = while {
            tunnel: w1074 -> [w1097]
            tunnel: w1073 -> [w1096]
            tunnel: [w1089] -> w1072
            tunnel: [w1088] -> w1071
            tunnel: w1076 -> [w1077]
            tunnel: w1075 -> [w1084]
            stop <- w1082 stop-if-true
            # "was 6000 counts"
            # "8,683.52 encoder counts to get to base line"
            n477 = global read "Robot Global Data.vi" "Left Encoder"() -> (w1085:dbl)
            n478 = global read "Robot Global Data.vi" "Right Encoder"() -> (w1087:dbl)
            n479 = call "inches to encoder counts.vi"("x inches"=30.0) -> ("encoder counts"=w1079:dbl)  [unwired: 10 in]
            n480 = Subtract(x=w1085, y=w1084) -> (x-y=w1083:dbl)
            n481 = Subtract(x=w1087, y=w1077) -> (x-y=w1086:dbl)
            n482 = Greater Or Equal?(x=w1086, y=w1079) -> (x >= y?=w1091:bool)
            n483 = Greater Or Equal?(x=w1083, y=w1079) -> (x >= y?=w1090:bool)
            n484 = Select(t=0.0, s=w1090, f=0.65) -> (s? t:f=w1080:dbl)
            n485 = Select(t=0.0, s=w1091, f=0.65) -> (s? t:f=w1081:dbl)
            n486 = And(x=w1091, y=w1090) -> (x .and. y?=w1082:bool)
            n487 = call <vilib>:"WPI_RobotDriveTankDrive.vi"("error in (no error)"=w1096, "Right axis value"=w1081, "Left axis value"=w1080, "RobotDriveDevRef"=w1097) -> ("error out"=w1088:errorcluster, "RobotDriveDevRef"=w1089:T3)  [unwired: 5 in, 1 out]
          }
        }
        frame #1 {
          n488 = while {
            tunnel: w1101 -> [w1102]
            tunnel: w1100 -> [w1103]
            tunnel: [w1105] -> w1099
            tunnel: [w1104] -> w1098
            stop <- w1106 continue-if-true
            # "use vision to drive to peg"
            n489 = call "Track peg with Pixy.vi"() -> ("sees peg"=w1106:bool, "y output"=w1107:dbl, "x output"=w1108:dbl)  [unwired: 8 in]
            n490 = call-poly <vilib>:"WPI_RobotDriveArcadeDrive.vi"("error in (no error)"=w1103, "Y axis value"=w1107, "X axis value"=w1108, "RobotDriveDevRef"=w1102) -> ("error out"=w1104:errorcluster, "RobotDriveDevRef"=w1105:T3)  [unwired: 5 in, 1 out]
          }
        }
        frame #2 {
          n491 = call-poly <vilib>:"WPI_RobotDriveArcadeDrive.vi"("error in (no error)"=w1112, "Y axis value"=0.4, "RobotDriveDevRef"=w1113) -> ("error out"=w1115:errorcluster, "RobotDriveDevRef"=w1116:T3)  [unwired: 6 in, 1 out]
          n492 = call <vilib>:"WPI_RobotDriveDelayAndUpdateSafety.vi"("error in (no error)"=w1115, "Delay (s)"=0.5, "RobotDriveDevRef"=w1116) -> ("error out"=w1110:errorcluster, "RobotDriveDevRef 2"=w1111:T3)  [unwired: 7 in]
        }
        frame #3 {
          # "unclamp gear"
          n493 = Tick Count (ms)() -> (millisecond timer value=w1119:u32)
          n494 = Add(x=w1119, y=u32 500) -> (x+y=w1118:u32)
          n495 = while {
            tunnel: w1118 -> [w1122]
            stop <- w1123 stop-if-true
            n496 = disable-structure shown="Enabled" {
              frame Enabled {
                n497 = call <vilib>:"WPI_RelayRefNum Registry Get.vi"("refnum name"="Gear Clamp") -> ("error out"=w1127:errorcluster, "RelayDevRef"=w1128:T8)  [unwired: 9 in]
                n498 = call <vilib>:"WPI_RelaySet.vi"("error in (no error)"=w1127, "RelayValue"=WPI_RelayValue."Reverse", "RelayDevRef"=w1128) -> ()  [unwired: 7 in, 2 out]
              }
              frame Disabled {
              }
            }
            n499 = Tick Count (ms)() -> (millisecond timer value=w1124:u32)
            n500 = Greater Or Equal?(x=w1124, y=w1122) -> (x >= y?=w1123:bool)
            "time up? 6" <- w1123
          }
        }
        frame #4 {
          # "set down gear"
          n501 = Tick Count (ms)() -> (millisecond timer value=w1131:u32)
          n502 = Add(x=w1131, y=u32 900) -> (x+y=w1129:u32)
          n503 = while {
            tunnel: w1129 -> [w1135]
            stop <- w1134 stop-if-true
            n504 = disable-structure shown="Enabled" {
              frame Enabled {
                n505 = call <vilib>:"WPI_RelayRefNum Registry Get.vi"("refnum name"="Gear Lift") -> ("error out"=w1139:errorcluster, "RelayDevRef"=w1140:T8)  [unwired: 9 in]
                n506 = call <vilib>:"WPI_RelaySet.vi"("error in (no error)"=w1139, "RelayValue"=WPI_RelayValue."Reverse", "RelayDevRef"=w1140) -> ()  [unwired: 7 in, 2 out]
              }
              frame Disabled {
              }
            }
            n507 = Tick Count (ms)() -> (millisecond timer value=w1136:u32)
            n508 = Greater Or Equal?(x=w1136, y=w1135) -> (x >= y?=w1134:bool)
            "time up? 5" <- w1134
          }
        }
        frame #5 {
          # "then backup for 1 sec"
          n509 = call-poly <vilib>:"WPI_RobotDriveArcadeDrive.vi"("error in (no error)"=w1141, "Y axis value"=-0.6, "RobotDriveDevRef"=w1142) -> ("error out"=w1145:errorcluster, "RobotDriveDevRef"=w1146:T3)  [unwired: 6 in, 1 out]
          n510 = call <vilib>:"WPI_RobotDriveDelayAndUpdateSafety.vi"("error in (no error)"=w1145, "Delay (s)"=1.0, "RobotDriveDevRef"=w1146) -> ()  [unwired: 7 in, 2 out]
        }
        frame #6 {
          n511 = call <vilib>:"WPI_RelayRefNum Registry Get.vi"("refnum name"="Gear Clamp") -> ("error out"=w1149:errorcluster, "RelayDevRef"=w1150:T8)  [unwired: 9 in]
          n512 = call <vilib>:"WPI_RelayRefNum Registry Get.vi"("refnum name"="Gear Lift") -> ("error out"=w1153:errorcluster, "RelayDevRef"=w1154:T8)  [unwired: 9 in]
          n513 = call <vilib>:"WPI_RelaySet.vi"("error in (no error)"=w1149, "RelayValue"=WPI_RelayValue."Off", "RelayDevRef"=w1150) -> ()  [unwired: 7 in, 2 out]
          n514 = call <vilib>:"WPI_RelaySet.vi"("error in (no error)"=w1153, "RelayValue"=WPI_RelayValue."Off", "RelayDevRef"=w1154) -> ()  [unwired: 7 in, 2 out]
        }
      }
    }
    frame "center peg shoot - right" {
      n515 = flat-sequence {
        tunnel: w1175 -> [w1178]
        tunnel: w1176 -> [w1179]
        tunnel: [w1179] -> w1158
        tunnel: [w1178] -> w1157
        tunnel: [w1181] -> w1166
        tunnel: [w1180] -> w1165
        tunnel: w1158 -> [w1183]
        tunnel: w1157 -> [w1182]
        tunnel: [w1208] -> w1168
        tunnel: [w1207] -> w1167
        tunnel: w1166 -> [w1210]
        tunnel: w1165 -> [w1209]
        tunnel: [w1220] -> w1174
        tunnel: [w1219] -> w1173
        tunnel: w1167 -> [w1221]
        tunnel: w1168 -> [w1222]
        tunnel: w1174 -> [w1226]
        tunnel: w1173 -> [w1230]
        tunnel: [w1226] -> w1172
        tunnel: [w1230] -> w1171
        tunnel: w1172 -> [w1242]
        tunnel: w1171 -> [w1241]
        tunnel: [w1242] -> w1170
        tunnel: [w1241] -> w1169
        tunnel: w1170 -> [w1253]
        tunnel: w1169 -> [w1252]
        tunnel: [w1251] -> w1163
        tunnel: [w1250] -> w1161
        tunnel: [w1276] -> w1164
        tunnel: w1163 -> [w1276]
        tunnel: [w1275] -> w1162
        tunnel: w1161 -> [w1275]
        tunnel: w1164 -> [w1289]
        tunnel: w1162 -> [w1287]
        tunnel: [w1286] -> w1160
        tunnel: [w1285] -> w1159
        tunnel: w1160 -> [w1293]
        tunnel: w1159 -> [w1292]
        tunnel: [w1291] -> w1156
        tunnel: [w1290] -> w1155
        tunnel: w1156 -> [w1317]
        tunnel: w1155 -> [w1316]
        frame #0 {
          n516 = global read "Robot Global Data.vi" "Navx fused heading"() -> (w1177:dbl)
          n517 = global write "Robot Global Data.vi" "Navx auto starting position"(w1177) -> ()
        }
        frame #1 {
          n518 = global read "Robot Global Data.vi" "Right Encoder"() -> (w1185:dbl)
          n519 = global read "Robot Global Data.vi" "Left Encoder"() -> (w1184:dbl)
          n520 = while {
            tunnel: w1183 -> [w1206]
            tunnel: w1182 -> [w1205]
            tunnel: [w1198] -> w1181
            tunnel: [w1197] -> w1180
            tunnel: w1185 -> [w1186]
            tunnel: w1184 -> [w1193]
            stop <- w1191 stop-if-true
            # "was 6000 counts"
            # "8,683.52 encoder counts to get to base line"
            n521 = global read "Robot Global Data.vi" "Left Encoder"() -> (w1194:dbl)
            n522 = global read "Robot Global Data.vi" "Right Encoder"() -> (w1196:dbl)
            n523 = call "inches to encoder counts.vi"("x inches"=30.0) -> ("encoder counts"=w1188:dbl)  [unwired: 10 in]
            n524 = Subtract(x=w1194, y=w1193) -> (x-y=w1192:dbl)
            n525 = Subtract(x=w1196, y=w1186) -> (x-y=w1195:dbl)
            n526 = Greater Or Equal?(x=w1195, y=w1188) -> (x >= y?=w1200:bool)
            n527 = Greater Or Equal?(x=w1192, y=w1188) -> (x >= y?=w1199:bool)
            n528 = Select(t=0.0, s=w1199, f=0.7) -> (s? t:f=w1189:dbl)
            n529 = Select(t=0.0, s=w1200, f=0.7) -> (s? t:f=w1190:dbl)
            n530 = And(x=w1200, y=w1199) -> (x .and. y?=w1191:bool)
            n531 = call <vilib>:"WPI_RobotDriveTankDrive.vi"("error in (no error)"=w1205, "Right axis value"=w1190, "Left axis value"=w1189, "RobotDriveDevRef"=w1206) -> ("error out"=w1197:errorcluster, "RobotDriveDevRef"=w1198:T3)  [unwired: 5 in, 1 out]
          }
        }
        frame #2 {
          n532 = while {
            tunnel: w1210 -> [w1211]
            tunnel: w1209 -> [w1212]
            tunnel: [w1214] -> w1208
            tunnel: [w1213] -> w1207
            stop <- w1215 continue-if-true
            # "use vision to drive to peg"
            n533 = call "Track peg with Pixy.vi"() -> ("sees peg"=w1215:bool, "y output"=w1216:dbl, "x output"=w1217:dbl)  [unwired: 8 in]
            n534 = call-poly <vilib>:"WPI_RobotDriveArcadeDrive.vi"("error in (no error)"=w1212, "Y axis value"=w1216, "X axis value"=w1217, "RobotDriveDevRef"=w1211) -> ("error out"=w1213:errorcluster, "RobotDriveDevRef"=w1214:T3)  [unwired: 5 in, 1 out]
          }
        }
        frame #3 {
          n535 = call-poly <vilib>:"WPI_RobotDriveArcadeDrive.vi"("error in (no error)"=w1221, "Y axis value"=0.35, "RobotDriveDevRef"=w1222) -> ("error out"=w1224:errorcluster, "RobotDriveDevRef"=w1225:T3)  [unwired: 6 in, 1 out]
          n536 = call <vilib>:"WPI_RobotDriveDelayAndUpdateSafety.vi"("error in (no error)"=w1224, "Delay (s)"=0.4, "RobotDriveDevRef"=w1225) -> ("error out"=w1219:errorcluster, "RobotDriveDevRef 2"=w1220:T3)  [unwired: 7 in]
        }
        frame #4 {
          # "unclamp gear"
          n537 = Tick Count (ms)() -> (millisecond timer value=w1228:u32)
          n538 = Add(x=w1228, y=u32 500) -> (x+y=w1227:u32)
          n539 = while {
            tunnel: w1227 -> [w1231]
            stop <- w1232 stop-if-true
            n540 = disable-structure shown="Enabled" {
              frame Enabled {
                n541 = call <vilib>:"WPI_RelayRefNum Registry Get.vi"("refnum name"="Gear Clamp") -> ("error out"=w1236:errorcluster, "RelayDevRef"=w1237:T8)  [unwired: 9 in]
                n542 = call <vilib>:"WPI_RelaySet.vi"("error in (no error)"=w1236, "RelayValue"=WPI_RelayValue."Reverse", "RelayDevRef"=w1237) -> ()  [unwired: 7 in, 2 out]
              }
              frame Disabled {
              }
            }
            n543 = Tick Count (ms)() -> (millisecond timer value=w1233:u32)
            n544 = Greater Or Equal?(x=w1233, y=w1231) -> (x >= y?=w1232:bool)
            "time up? 13" <- w1232
          }
        }
        frame #5 {
          # "set down gear"
          n545 = Tick Count (ms)() -> (millisecond timer value=w1240:u32)
          n546 = Add(x=w1240, y=u32 900) -> (x+y=w1238:u32)
          n547 = while {
            tunnel: w1238 -> [w1244]
            stop <- w1243 stop-if-true
            n548 = disable-structure shown="Enabled" {
              frame Enabled {
                n549 = call <vilib>:"WPI_RelayRefNum Registry Get.vi"("refnum name"="Gear Lift") -> ("error out"=w1248:errorcluster, "RelayDevRef"=w1249:T8)  [unwired: 9 in]
                n550 = call <vilib>:"WPI_RelaySet.vi"("error in (no error)"=w1248, "RelayValue"=WPI_RelayValue."Reverse", "RelayDevRef"=w1249) -> ()  [unwired: 7 in, 2 out]
              }
              frame Disabled {
              }
            }
            n551 = Tick Count (ms)() -> (millisecond timer value=w1245:u32)
            n552 = Greater Or Equal?(x=w1245, y=w1244) -> (x >= y?=w1243:bool)
            "time up? 14" <- w1243
          }
        }
        frame #6 {
          n553 = global read "Robot Global Data.vi" "Right Encoder"() -> (w1255:dbl)
          n554 = global read "Robot Global Data.vi" "Left Encoder"() -> (w1254:dbl)
          n555 = while {
            tunnel: w1253 -> [w1274]
            tunnel: w1252 -> [w1273]
            tunnel: [w1272] -> w1251
            tunnel: [w1271] -> w1250
            tunnel: w1255 -> [w1269]
            tunnel: w1254 -> [w1267]
            stop <- w1257 continue-if-true
            n556 = global read "Robot Global Data.vi" "Left Encoder"() -> (w1268:dbl)
            n557 = global read "Robot Global Data.vi" "Right Encoder"() -> (w1270:dbl)
            n558 = Subtract(x=w1268, y=w1267) -> (x-y=w1264:dbl)
            n559 = Subtract(x=w1270, y=w1269) -> (x-y=w1265:dbl)
            n560 = Add(x=w1265, y=w1264) -> (x+y=w1263:dbl)
            n561 = Divide(x=w1263, y=2.0) -> (x/y=w1259:dbl)
            n562 = call "inches to encoder counts.vi"("x inches"=-18.0) -> ("encoder counts"=w1260:dbl)  [unwired: 10 in]
            n563 = Less?(x=w1260, y=w1259) -> (x < y?=w1257:bool)
            n564 = Select(t=-0.55, s=w1257, f=0.0) -> (s? t:f=w1256:dbl)
            n565 = call-poly <vilib>:"WPI_RobotDriveArcadeDrive.vi"("error in (no error)"=w1273, "Y axis value"=w1256, "RobotDriveDevRef"=w1274) -> ("error out"=w1271:errorcluster, "RobotDriveDevRef"=w1272:T3)  [unwired: 6 in, 1 out]
          }
        }
        frame #7 {
          n566 = call <vilib>:"WPI_RelayRefNum Registry Get.vi"("refnum name"="Gear Clamp") -> ("error out"=w1279:errorcluster, "RelayDevRef"=w1280:T8)  [unwired: 9 in]
          n567 = call <vilib>:"WPI_RelayRefNum Registry Get.vi"("refnum name"="Gear Lift") -> ("error out"=w1283:errorcluster, "RelayDevRef"=w1284:T8)  [unwired: 9 in]
          n568 = call <vilib>:"WPI_RelaySet.vi"("error in (no error)"=w1279, "RelayValue"=WPI_RelayValue."Off", "RelayDevRef"=w1280) -> ()  [unwired: 7 in, 2 out]
          n569 = call <vilib>:"WPI_RelaySet.vi"("error in (no error)"=w1283, "RelayValue"=WPI_RelayValue."Off", "RelayDevRef"=w1284) -> ()  [unwired: 7 in, 2 out]
        }
        frame #8 {
          # "was -80 then 76"
          n570 = call "example use of turn power block.vi"("error in (no error)"=w1287, "desired angle"=-72.0, "RobotDriveDevRef"=w1289) -> ("error out"=w1285:errorcluster, "RobotDriveDevRef 2"=w1286:T3)  [unwired: 7 in]
        }
        frame #9 {
          n571 = global read "Robot Global Data.vi" "Right Encoder"() -> (w1295:dbl)
          n572 = global read "Robot Global Data.vi" "Left Encoder"() -> (w1294:dbl)
          n573 = while {
            tunnel: w1293 -> [w1314]
            tunnel: w1292 -> [w1313]
            tunnel: [w1312] -> w1291
            tunnel: [w1311] -> w1290
            tunnel: w1295 -> [w1309]
            tunnel: w1294 -> [w1307]
            stop <- w1297 continue-if-true
            n574 = global read "Robot Global Data.vi" "Left Encoder"() -> (w1308:dbl)
            n575 = global read "Robot Global Data.vi" "Right Encoder"() -> (w1310:dbl)
            n576 = Subtract(x=w1308, y=w1307) -> (x-y=w1304:dbl)
            n577 = Subtract(x=w1310, y=w1309) -> (x-y=w1305:dbl)
            n578 = Add(x=w1305, y=w1304) -> (x+y=w1303:dbl)
            n579 = Divide(x=w1303, y=2.0) -> (x/y=w1299:dbl)
            n580 = call "inches to encoder counts.vi"("x inches"=-50.0) -> ("encoder counts"=w1300:dbl)  [unwired: 10 in]
            n581 = Less?(x=w1300, y=w1299) -> (x < y?=w1297:bool)
            n582 = Select(t=-0.7, s=w1297, f=0.0) -> (s? t:f=w1296:dbl)
            n583 = call-poly <vilib>:"WPI_RobotDriveArcadeDrive.vi"("error in (no error)"=w1313, "Y axis value"=w1296, "RobotDriveDevRef"=w1314) -> ("error out"=w1311:errorcluster, "RobotDriveDevRef"=w1312:T3)  [unwired: 6 in, 1 out]
          }
        }
        frame #10 {
          n584 = call "shoot boiler.vi"("go"=TRUE, "error out"=w1316, "RobotDriveDevRef"=w1317) -> ()  [unwired: 7 in, 2 out]
        }
      }
    }
    frame "center peg shoot - left" {
      n585 = flat-sequence {
        tunnel: w1338 -> [w1341]
        tunnel: w1339 -> [w1342]
        tunnel: [w1342] -> w1321
        tunnel: [w1341] -> w1320
        tunnel: [w1344] -> w1329
        tunnel: [w1343] -> w1328
        tunnel: w1321 -> [w1346]
        tunnel: w1320 -> [w1345]
        tunnel: [w1371] -> w1331
        tunnel: [w1370] -> w1330
        tunnel: w1329 -> [w1373]
        tunnel: w1328 -> [w1372]
        tunnel: [w1383] -> w1337
        tunnel: [w1382] -> w1336
        tunnel: w1330 -> [w1384]
        tunnel: w1331 -> [w1385]
        tunnel: w1337 -> [w1389]
        tunnel: w1336 -> [w1393]
        tunnel: [w1389] -> w1335
        tunnel: [w1393] -> w1334
        tunnel: w1335 -> [w1405]
        tunnel: w1334 -> [w1404]
        tunnel: [w1405] -> w1333
        tunnel: [w1404] -> w1332
        tunnel: w1333 -> [w1416]
        tunnel: w1332 -> [w1415]
        tunnel: [w1414] -> w1326
        tunnel: [w1413] -> w1324
        tunnel: [w1439] -> w1327
        tunnel: w1326 -> [w1439]
        tunnel: [w1438] -> w1325
        tunnel: w1324 -> [w1438]
        tunnel: w1327 -> [w1452]
        tunnel: w1325 -> [w1450]
        tunnel: [w1449] -> w1323
        tunnel: [w1448] -> w1322
        tunnel: w1323 -> [w1456]
        tunnel: w1322 -> [w1455]
        tunnel: [w1454] -> w1319
        tunnel: [w1453] -> w1318
        tunnel: w1319 -> [w1480]
        tunnel: w1318 -> [w1479]
        frame #0 {
          n586 = global read "Robot Global Data.vi" "Navx fused heading"() -> (w1340:dbl)
          n587 = global write "Robot Global Data.vi" "Navx auto starting position"(w1340) -> ()
        }
        frame #1 {
          n588 = global read "Robot Global Data.vi" "Right Encoder"() -> (w1348:dbl)
          n589 = global read "Robot Global Data.vi" "Left Encoder"() -> (w1347:dbl)
          n590 = while {
            tunnel: w1346 -> [w1369]
            tunnel: w1345 -> [w1368]
            tunnel: [w1361] -> w1344
            tunnel: [w1360] -> w1343
            tunnel: w1348 -> [w1349]
            tunnel: w1347 -> [w1356]
            stop <- w1354 stop-if-true
            # "was 6000 counts"
            # "8,683.52 encoder counts to get to base line"
            n591 = global read "Robot Global Data.vi" "Left Encoder"() -> (w1357:dbl)
            n592 = global read "Robot Global Data.vi" "Right Encoder"() -> (w1359:dbl)
            n593 = call "inches to encoder counts.vi"("x inches"=30.0) -> ("encoder counts"=w1351:dbl)  [unwired: 10 in]
            n594 = Subtract(x=w1357, y=w1356) -> (x-y=w1355:dbl)
            n595 = Subtract(x=w1359, y=w1349) -> (x-y=w1358:dbl)
            n596 = Greater Or Equal?(x=w1358, y=w1351) -> (x >= y?=w1363:bool)
            n597 = Greater Or Equal?(x=w1355, y=w1351) -> (x >= y?=w1362:bool)
            n598 = Select(t=0.0, s=w1362, f=0.7) -> (s? t:f=w1352:dbl)
            n599 = Select(t=0.0, s=w1363, f=0.7) -> (s? t:f=w1353:dbl)
            n600 = And(x=w1363, y=w1362) -> (x .and. y?=w1354:bool)
            n601 = call <vilib>:"WPI_RobotDriveTankDrive.vi"("error in (no error)"=w1368, "Right axis value"=w1353, "Left axis value"=w1352, "RobotDriveDevRef"=w1369) -> ("error out"=w1360:errorcluster, "RobotDriveDevRef"=w1361:T3)  [unwired: 5 in, 1 out]
          }
        }
        frame #2 {
          n602 = while {
            tunnel: w1373 -> [w1374]
            tunnel: w1372 -> [w1375]
            tunnel: [w1377] -> w1371
            tunnel: [w1376] -> w1370
            stop <- w1378 continue-if-true
            # "use vision to drive to peg"
            n603 = call "Track peg with Pixy.vi"() -> ("sees peg"=w1378:bool, "y output"=w1379:dbl, "x output"=w1380:dbl)  [unwired: 8 in]
            n604 = call-poly <vilib>:"WPI_RobotDriveArcadeDrive.vi"("error in (no error)"=w1375, "Y axis value"=w1379, "X axis value"=w1380, "RobotDriveDevRef"=w1374) -> ("error out"=w1376:errorcluster, "RobotDriveDevRef"=w1377:T3)  [unwired: 5 in, 1 out]
          }
        }
        frame #3 {
          n605 = call-poly <vilib>:"WPI_RobotDriveArcadeDrive.vi"("error in (no error)"=w1384, "Y axis value"=0.35, "RobotDriveDevRef"=w1385) -> ("error out"=w1387:errorcluster, "RobotDriveDevRef"=w1388:T3)  [unwired: 6 in, 1 out]
          n606 = call <vilib>:"WPI_RobotDriveDelayAndUpdateSafety.vi"("error in (no error)"=w1387, "Delay (s)"=0.4, "RobotDriveDevRef"=w1388) -> ("error out"=w1382:errorcluster, "RobotDriveDevRef 2"=w1383:T3)  [unwired: 7 in]
        }
        frame #4 {
          # "unclamp gear"
          n607 = Tick Count (ms)() -> (millisecond timer value=w1391:u32)
          n608 = Add(x=w1391, y=u32 500) -> (x+y=w1390:u32)
          n609 = while {
            tunnel: w1390 -> [w1394]
            stop <- w1395 stop-if-true
            n610 = disable-structure shown="Enabled" {
              frame Enabled {
                n611 = call <vilib>:"WPI_RelayRefNum Registry Get.vi"("refnum name"="Gear Clamp") -> ("error out"=w1399:errorcluster, "RelayDevRef"=w1400:T8)  [unwired: 9 in]
                n612 = call <vilib>:"WPI_RelaySet.vi"("error in (no error)"=w1399, "RelayValue"=WPI_RelayValue."Reverse", "RelayDevRef"=w1400) -> ()  [unwired: 7 in, 2 out]
              }
              frame Disabled {
              }
            }
            n613 = Tick Count (ms)() -> (millisecond timer value=w1396:u32)
            n614 = Greater Or Equal?(x=w1396, y=w1394) -> (x >= y?=w1395:bool)
            "time up? 15" <- w1395
          }
        }
        frame #5 {
          # "set down gear"
          n615 = Tick Count (ms)() -> (millisecond timer value=w1403:u32)
          n616 = Add(x=w1403, y=u32 900) -> (x+y=w1401:u32)
          n617 = while {
            tunnel: w1401 -> [w1407]
            stop <- w1406 stop-if-true
            n618 = disable-structure shown="Enabled" {
              frame Enabled {
                n619 = call <vilib>:"WPI_RelayRefNum Registry Get.vi"("refnum name"="Gear Lift") -> ("error out"=w1411:errorcluster, "RelayDevRef"=w1412:T8)  [unwired: 9 in]
                n620 = call <vilib>:"WPI_RelaySet.vi"("error in (no error)"=w1411, "RelayValue"=WPI_RelayValue."Reverse", "RelayDevRef"=w1412) -> ()  [unwired: 7 in, 2 out]
              }
              frame Disabled {
              }
            }
            n621 = Tick Count (ms)() -> (millisecond timer value=w1408:u32)
            n622 = Greater Or Equal?(x=w1408, y=w1407) -> (x >= y?=w1406:bool)
            "time up? 16" <- w1406
          }
        }
        frame #6 {
          n623 = global read "Robot Global Data.vi" "Right Encoder"() -> (w1418:dbl)
          n624 = global read "Robot Global Data.vi" "Left Encoder"() -> (w1417:dbl)
          n625 = while {
            tunnel: w1416 -> [w1437]
            tunnel: w1415 -> [w1436]
            tunnel: [w1435] -> w1414
            tunnel: [w1434] -> w1413
            tunnel: w1418 -> [w1432]
            tunnel: w1417 -> [w1430]
            stop <- w1420 continue-if-true
            n626 = global read "Robot Global Data.vi" "Left Encoder"() -> (w1431:dbl)
            n627 = global read "Robot Global Data.vi" "Right Encoder"() -> (w1433:dbl)
            n628 = Subtract(x=w1431, y=w1430) -> (x-y=w1427:dbl)
            n629 = Subtract(x=w1433, y=w1432) -> (x-y=w1428:dbl)
            n630 = Add(x=w1428, y=w1427) -> (x+y=w1426:dbl)
            n631 = Divide(x=w1426, y=2.0) -> (x/y=w1422:dbl)
            n632 = call "inches to encoder counts.vi"("x inches"=-18.0) -> ("encoder counts"=w1423:dbl)  [unwired: 10 in]
            n633 = Less?(x=w1423, y=w1422) -> (x < y?=w1420:bool)
            n634 = Select(t=-0.55, s=w1420, f=0.0) -> (s? t:f=w1419:dbl)
            n635 = call-poly <vilib>:"WPI_RobotDriveArcadeDrive.vi"("error in (no error)"=w1436, "Y axis value"=w1419, "RobotDriveDevRef"=w1437) -> ("error out"=w1434:errorcluster, "RobotDriveDevRef"=w1435:T3)  [unwired: 6 in, 1 out]
          }
        }
        frame #7 {
          n636 = call <vilib>:"WPI_RelayRefNum Registry Get.vi"("refnum name"="Gear Clamp") -> ("error out"=w1442:errorcluster, "RelayDevRef"=w1443:T8)  [unwired: 9 in]
          n637 = call <vilib>:"WPI_RelayRefNum Registry Get.vi"("refnum name"="Gear Lift") -> ("error out"=w1446:errorcluster, "RelayDevRef"=w1447:T8)  [unwired: 9 in]
          n638 = call <vilib>:"WPI_RelaySet.vi"("error in (no error)"=w1442, "RelayValue"=WPI_RelayValue."Off", "RelayDevRef"=w1443) -> ()  [unwired: 7 in, 2 out]
          n639 = call <vilib>:"WPI_RelaySet.vi"("error in (no error)"=w1446, "RelayValue"=WPI_RelayValue."Off", "RelayDevRef"=w1447) -> ()  [unwired: 7 in, 2 out]
        }
        frame #8 {
          n640 = call "example use of turn power block.vi"("error in (no error)"=w1450, "desired angle"=72.0, "RobotDriveDevRef"=w1452) -> ("error out"=w1448:errorcluster, "RobotDriveDevRef 2"=w1449:T3)  [unwired: 7 in]
        }
        frame #9 {
          n641 = global read "Robot Global Data.vi" "Right Encoder"() -> (w1458:dbl)
          n642 = global read "Robot Global Data.vi" "Left Encoder"() -> (w1457:dbl)
          n643 = while {
            tunnel: w1456 -> [w1477]
            tunnel: w1455 -> [w1476]
            tunnel: [w1475] -> w1454
            tunnel: [w1474] -> w1453
            tunnel: w1458 -> [w1472]
            tunnel: w1457 -> [w1470]
            stop <- w1460 continue-if-true
            n644 = global read "Robot Global Data.vi" "Left Encoder"() -> (w1471:dbl)
            n645 = global read "Robot Global Data.vi" "Right Encoder"() -> (w1473:dbl)
            n646 = Subtract(x=w1471, y=w1470) -> (x-y=w1467:dbl)
            n647 = Subtract(x=w1473, y=w1472) -> (x-y=w1468:dbl)
            n648 = Add(x=w1468, y=w1467) -> (x+y=w1466:dbl)
            n649 = Divide(x=w1466, y=2.0) -> (x/y=w1462:dbl)
            n650 = call "inches to encoder counts.vi"("x inches"=-50.0) -> ("encoder counts"=w1463:dbl)  [unwired: 10 in]
            n651 = Less?(x=w1463, y=w1462) -> (x < y?=w1460:bool)
            n652 = Select(t=-0.7, s=w1460, f=0.0) -> (s? t:f=w1459:dbl)
            n653 = call-poly <vilib>:"WPI_RobotDriveArcadeDrive.vi"("error in (no error)"=w1476, "Y axis value"=w1459, "RobotDriveDevRef"=w1477) -> ("error out"=w1474:errorcluster, "RobotDriveDevRef"=w1475:T3)  [unwired: 6 in, 1 out]
          }
        }
        frame #10 {
          n654 = call "shoot boiler.vi"("go"=TRUE, "error out"=w1479, "RobotDriveDevRef"=w1480) -> ()  [unwired: 7 in, 2 out]
        }
      }
    }
  }
